vi "Text control 2 v5.1_pump-specific.vi"() -> ()   [LabVIEW 2016]
panel:
  in  "Tab Control":enum32{"Main", "Other parameters"}(tab)
  out "Line running":i32
  out "Total lines":i32
  out "Path":path=path "C:/users/rlp38/09Apr2009LTtesting/test2.txt"
  out "I vs Vg":cluster{"Y data in":dbl[], "X data in":dbl[]}[](graph)
  out "Is max":dbl format="%.2e"
  out "Id max":dbl format="%.2e"
  out "Ig max":dbl format="%.2e"
  out "Imax vs time":cluster{"Y data in":dbl[], "X data in":dbl[]}[](graph)
  out "Imin vs time":cluster{"Y data in":dbl[], "X data in":dbl[]}[](graph)
  out "I vs Vd":cluster{"Y data in":dbl[], "X data in":dbl[]}[](graph)
  in  "Program":string="#-------------------------------------------------------\n# Priming script\n#\n# Version 0.5\n# Author: Dimitrios Simatos\n# Last updated: 2017-10-17\n#-------------------------------------------------------\n# Description\n#\n# This script is designed to prime inlet ports 3, 5 and outlet port 2.\n#-------------------------------------------------------\n# Changes\n#\n# Replaced instances of counterclockwise with clockwise rotation.\n#-------------------------------------------------------\n# Important points\n#\n# Never leave any liquid in the pump to dry after the experiments. If they dry, the residue may block the valve.\n# Always run the cleaning cycle after the experiments.\n# Use clockwise rotation when going up in valve port numbers and vice versa.\n#-------------------------------------------------------\n# Things to do before running the script\n#\n# Set time units to minutes.\n# Set filenames.\n# Replace the tubing, if necessary.\n#-------------------------------------------------------\n# Port connections\n#\n# Port 1: Waste\n# Port 2: Waste\n# Port 3: Ultrapure water\n# Port 4: Nothing\n# Port 5: Phosphate buffer (pH=3.2 - 50 mM)\n# Port 6: Nothing\n#-------------------------------------------------------\n# Pumping cycles and execution time\n#\n# Execution time: 4 x 2 = 8 minutes\n# Ultrapure water must be the last to be pumped through the valve, to wash away residual ions.\n# There are 4 pumping cycles. The first two are small, priming cycles, and the last two are large, cleaning and priming cycles.\n# Each small pumping cycle primes the tubing of each port.\n# The last two cycle prime the tubing of the port containing ultrapure water (port 3) and also pump it through the valve, to clean the valve, the syringe, and prime the tubing of the device port (port 2).\n# The device must be disconnected from the port during the priming procedure.\n#-------------------------------------------------------\n# Volume of liquid needed\n#\n# Volume of liquid needed per small cycle: 200 ul\n# Volume of liquid needed per large cycle: 800 ul\n# Total volume of liquid needed per script run:\n# 200 ul of phosphate buffer (pH=3.2 - 50 mM)\n# 200 + 2 x 800 = 1800 ul of ultrapure water\n#-------------------------------------------------------\n# Parameters\n#\n# Syringe size: 1 ml\n# Step resolution N = 0.01 mm\n# Flow V = 300 pulses/second (6000 ul/min)\n#-------------------------------------------------------\n# Cycle 1: Priming the tubing of the phosphate buffer (pH=3.2 - 50 mM) port (port 5)\npump /1ZR #initialize pump\npump /1Q #query pump\npump /1? #report absolute plunger position\n#pump /1?6 #report valve position\nwait-min 1 #wait 1 minute\npump /1N0R #set step resolution: 0.01 mm\npump /1Q #query pump\npump /1? #report absolute plunger position (the plunger should be at 0)\npump /1?6 #report valve position\nwait 1000 #wait 1 second\npump /1V300R #choose speed: 300 steps/s\npump /1Q #query pump\nwait 1000 #wait 1 second\npump /1O5R #go to port 5, counterclockwise rotation\npump /1Q #query pump\npump /1?6 #report valve position\nwait 1000 #wait 1 second\npump /1A600R #go to absolute position 600 (= draw 200 ul)\n# The position of the plunger depends on the volume of the tubing. The syringe must draw enough liquid to fill the tubing.\nwait 30000 #wait 30 seconds\npump /1Q #query pump\npump /1? #report absolute plunger position (the plunger should have finished moving)\n#pump /1?6 #report valve position\npump /1I1R #switch to port 1, clockwise rotation\npump /1Q #query pump\npump /1?6 #report valve position\npump /1A0R #go to absolute position 0 (= empty syringe)\npump /1Q #query pump\npump /1? #report absolute plunger position (the plunger should be moving to 0)\n#pump /1?6 #report valve position\nwait-min 1 #wait 1 minute\n#-------------------------------------------------------\n# Cycle 2: Priming the tubing of the ultrapure water port (port 3)\n#pump /1ZR #initialize pump\npump /1Q #query pump\npump /1? #report absolute plunger position\npump /1?6 #report valve position\nwait-min 1 #wait 1 minute\npump /1N0R #set step resolution: 0.01 mm\npump /1Q #query pump\npump /1? #report absolute plunger position (the plunger should be at 0)\npump /1?6 #report valve position\nwait 1000 #wait 1 second\npump /1V300R #choose speed: 300 steps/s\npump /1Q #query pump\nwait 1000 #wait 1 second\npump /1I3R #go to port 3, clockwise rotation\npump /1Q #query pump\npump /1?6 #report valve position\nwait 1000 #wait 1 second\npump /1A600R #go to absolute position 600 (= draw 200 ul)\n# The position of the plunger depends on the volume of the tubing. The syringe must draw enough liquid to fill the tubing.\nwait 30000 #wait 30 seconds\npump /1Q #query pump\npump /1? #report absolute plunger position (the plunger should have finished moving)\n#pump /1?6 #report valve position\npump /1O1R #switch to port 1, counterclockwise rotation\npump /1Q #query pump\npump /1?6 #report valve position\npump /1A0R #go to absolute position 0 (= empty syringe)\npump /1Q #query pump\npump /1?6 #report valve position\npump /1? #report absolute plunger position (the plunger should be moving to 0)\n#pump /1?6 #report valve position\nwait-min 1 #wait 1 minute\n#-------------------------------------------------------\n# Cycle 3: Cleaning the syringe and the tubing of device port (port 2) (1/2)\n#pump /1ZR #initialize pump\npump /1Q #query pump\npump /1? #report absolute plunger position\npump /1?6 #report valve position\nwait-min 1 #wait 1 minute\npump /1N0R #set step resolution: 0.01 mm\npump /1Q #query pump\npump /1? #report absolute plunger position (the plunger should be at 0)\npump /1?6 #report valve position\nwait 1000 #wait 1 second\npump /1V300R #choose speed: 300 steps/s\npump /1Q #query pump\nwait 1000 #wait 1 second\npump /1I3R #go to port 3, clockwise rotation\npump /1Q #query pump\npump /1?6 #report valve position\nwait 1000 #wait 1 second\npump /1A2400R #go to absolute position 2400 (= draw 800 ul)\n# The position of the plunger depends on the volume of the tubing. The syringe must draw enough liquid to fill the tubing.\nwait 30000 #wait 30 seconds\npump /1Q #query pump\npump /1? #report absolute plunger position (the plunger should have finished moving)\n#pump /1?6 #report valve position\npump /1O2R #switch to port 2, counterclockwise rotation\npump /1Q #query pump\npump /1?6 #report valve position\npump /1A0R #go to absolute position 0 (= empty syringe)\npump /1Q #query pump\npump /1? #report absolute plunger position (the plunger should be moving to 0)\n#pump /1?6 #report valve position\nwait-min 1 #wait 1 minute\n#-------------------------------------------------------\n# Cycle 4: Cleaning the syringe and the tubing of device port (port 2) (2/2)\n#pump /1ZR #initialize pump\npump /1Q #query pump\npump /1? #report absolute plunger position\npump /1?6 #report valve position\nwait-min 1 #wait 1 minute\npump /1N0R #set step resolution: 0.01 mm\npump /1Q #query pump\npump /1? #report absolute plunger position (the plunger should be at 0)\npump /1?6 #report valve position\nwait 1000 #wait 1 second\npump /1V300R #choose speed: 300 steps/s\npump /1Q #query pump\nwait 1000 #wait 1 second\npump /1I3R #go to port 3, clockwise rotation\npump /1Q #query pump\npump /1?6 #report valve position\nwait 1000 #wait 1 second\npump /1A2400R #go to absolute position 2400 (= draw 800 ul)\n# The position of the plunger depends on the volume of the tubing. The syringe must draw enough liquid to fill the tubing.\nwait 30000 #wait 30 seconds\npump /1Q #query pump\npump /1? #report absolute plunger position (the plunger should have finished moving)\n#pump /1?6 #report valve position\npump /1O2R #switch to port 2, counterclockwise rotation\npump /1Q #query pump\npump /1?6 #report valve position\npump /1A0R #go to absolute position 0 (= empty syringe)\npump /1Q #query pump\npump /1? #report absolute plunger position (the plunger should be moving to 0)\n#pump /1?6 #report valve position\nwait-min 1 #wait 1 minute\n#-------------------------------------------------------"
  out "Command running:":string
  out "Serial port data":string
  out "Elapsed Time":dbl caption="Elapsed Time (s)"
  in  "Units":u16(ring)=1 items=["Seconds", "Minutes", "Hours"]
  in  "Time Offset":dbl caption="Set Start Time (s)"
  in  "Reset":bool
  in  "Auto Reset":bool
  in  "integration time":u32(slide) max=2 step=1 scale=0.0..2.0
  in  "Interrupt run":bool
  out "Absolute plunger position vs time":cluster{"Y data in":dbl[], "X data in":dbl[]}[](graph)
  out "Valve position vs time":cluster{"Y data in":dbl[], "X data in":dbl[]}[](graph)
  in  "Halt pump":bool
  in  "Hard stop pump":bool
  out "Is on":dbl format="%.2e"
  out "Id on":dbl format="%.2e"
  out "Ig on":dbl format="%.2e"
  out "Ion vs time":cluster{"Y data in":dbl[], "X data in":dbl[]}[](graph)
  out "Ioff vs time":cluster{"Y data in":dbl[], "X data in":dbl[]}[](graph)
  out "Ig min":dbl format="%.2e"
  out "Id min":dbl format="%.2e"
  out "Is min":dbl format="%.2e"
  out "Is off":dbl format="%.2e"
  out "Id off":dbl format="%.2e"
  out "Ig off":dbl format="%.2e"
  in  "Gate Range\nmode":u16(ring) items=["Auto", "Limited", "Fixed"]
  in  "Gate Range":u8(slide)=6 max=11 scale=0.0..11.0
  in  "Source/Drain\nRange mode":u16(ring) items=["Auto", "Limited", "Fixed"]
  in  "Source/Drain Range":u8(slide)=6 max=11 scale=0.0..11.0
  in  "Panel Controls":T1={"Emergency Stop"=refnum, "TransGraph Max"=1e-05, "Text/Graph (text=false)"=TRUE} {"TransGraph Max" format="%.2e"}
  in  "Panel Controls 2":T2={"Emergency Stop"=refnum, "TransGraph Max"=1e-05, "Text/Graph (text=false)"=TRUE, "TransGraph Min"=1e-11} {"TransGraph Min" format="%.2e"; "TransGraph Max" format="%.2e"}
  in  "SMU4":cluster{"on/off":bool, "Voltage":dbl} {"Voltage" min=-100.0 max=100.0 format="%.2f"}
  in  "Full Reset":bool
  in  "Standby":T3
  out "error out":errorcluster
  in  "Delay before read (ms)":u32=1000
  in  "byte count":u32=64
  in  "Serial End Mode for Reads":u16(ring)=2 items=["None", "LastBit", "TermChar"]
  in  "Timeout (ms)":u32=10000
  in  "Enable Termination\nChar (T)":bool=TRUE
  in  "Termination char\n(0xA = '\\n' = LF)\n(0xD = '\\r' = CR)":u8=13 format="%.0x"
  in  "flow control":u16(ring) items=["None"=0, "XON/XOFF"=1, "RTS/CTS"=2, "DTR/DSR"=4]
  in  "stop bits":u16(ring)=10 items=["1.0"=10, "1.5"=15, "2.0"=20]
  in  "parity":u16(ring) items=["None", "Odd", "Even", "Mark", "Space"]
  in  "data bits":u16=8 min=5 max=8 step=1
  in  "VISA resource name":refnum<visa-resource-name>="COM6"
  in  "baud rate":u32=9600
  in  "Drain: Compliance":dbl=0.001 format="%.8f"
  in  "Gate: Compliance":dbl=0.001 format="%.8f"
  in  "hold time /s":dbl format="%.2f"
  in  "delay time /s":dbl format="%.2f"
  in  "Integration time (short)":dbl=0.0019 min=8e-05 max=0.0019 step=8e-05 format="%^.0e"
  in  "Integration time (long)":dbl=0.32 min=0.04 max=2.0 step=0.02 format="%.2f"
  in  "Step delay /s":dbl format="%.2f"
  in  "Prefix (transfer)":string="_step_1_ultrapure_H2O_"
  in  "Suffix (transfer)":string="_T.txt"
  in  "Prefix (Imax,Imin,Ion,Ioff)":string="_step_1_ultrapure_H2O_Imax_Imin_Ion_Ioff_vs_time"
  in  "Suffix (Idmax-Idmin)":string=".txt"
  in  "Prefix (output)":string="_step_1_ultrapure_H2O_"
  in  "Suffix (output)":string="_O.txt"
  in  "Prefix (script)":string="_step_1_ultrapure_H2O_script"
  in  "Prefix (serial port log)":string="_step_1_ultrapure_H2O_serial port output"
  in  "Prefix (plunger)":string="_step_1_ultrapure_H2O_plunger_vs_time"
  in  "Suffix (plunger)":string=".txt"
  in  "Prefix (valve)":string="_step_1_ultrapure_H2O_valve_port_vs_time"
  in  "Suffix (valve)":string=".txt"
  in  "Gate":T4={"Gate Start"=0.0, "Gate Stop"=2.0, "Gate Step (linear only)"=1.0, "Gate Compliance"=0.0001, "Gate PComp"=0.0, "Range mode"=0, "Range"=6} {"Range" max=11 scale=0.0..11.0; "Range mode" items=["Auto", "Limited", "Fixed"]; "Gate PComp" format="%^.2e"; "Gate Compliance" format="%^.2e"; "Gate Step (linear only)" format="%^.4e"; "Gate Stop" format="%^.4e"; "Gate Start" format="%^.4e"}
  in  "Drain 2":T5={"Drain Start"=0.0, "Drain Stop"=2.0, "Drain Compliance"=0.0001, "Drain Step"=1.0, "Drain PComp"=0.0, "Range mode"=0, "Range"=6} {"Range" max=11 scale=0.0..11.0; "Range mode" items=["Auto", "Limited", "Fixed"]; "Drain PComp" format="%^.2e"; "Drain Step" format="%^.4e"; "Drain Compliance" format="%^.2e"; "Drain Stop" format="%^.4e"; "Drain Start" format="%^.4e"}
  in  "Timings 2":T6={"integration time"=0, "Short/Long integration time"=0.00064, "hold time (sec)"=0.0, "delay time (sec)"=0.0, "Step Time (0 disables)"=0.0, "sweep method"=0, "Pulse period"=0.005, "Base voltage"=0.0, "Pulse width"=0.0005} {"Pulse width" min=0.0005 max=0.1 step=0.0001 format="%.4f"; "Base voltage" format="%^.4e"; "Pulse period" min=0.005 max=1.0 step=0.0001 format="%.4f"; "sweep method" items=["Continuous", "Pulsed"]; "Step Time (0 disables)" format="%.2f"; "delay time (sec)" format="%.4f"; "hold time (sec)" format="%.4f"; "Short/Long integration time" format="%^.0e"; "integration time" scale=0.0..2.0}
  # "Syntax:\nitime [s|m|l]\ngaterangemode [a|l|f]\ndrainrangemode [a|l|f]\npulsed [on|off] PulsePeriod(sec) PulseBaseVoltage PulseONWidth(sec)\nstandby [on l off]\nwait NumMilliseconds\nwait-min NumMinutes\n# texthere = comment\ntransfer [s|d] VgStart VgStop VgStep VdStart VdStop VdStep\noutput [s|d] VgStart VgStop VgStep VdStart VdStop VdStep\nsample Vg Vd NumSamples Time(s) SampleInterval(s)\nsamplei Idg NumSamples Time(s) SampleInterval(s) VDGcompliance\n100 samples is approximately 13 seconds with medium integration\n# if in doubt use SampleInterval(s) = 0.004\nstressV VG VD IGcompliance IDcompliance Duration(sec)\nstressI IDG VDGcompliance Duration(sec)\nvsu2pulse Bias Duration(s)\npulsedstressV [s|d] VEstop VgON VgOFF Period(s) PulseONwidth(s) Vd\nsample-fpp Vg Vd NumSamples Time\nresample-fpp Vg Vd\ntransfer-fpp [s|d] VgStart VgStop VgStep VdStart VdStop VdStep\noutput-fpp [s|d] VgStart VgStop VgStep VdStart VdStop VdStep\nserial SerialPortCommand\npump SerialPortCommand for the OEM pump\n\nSPM OEM Pump Syntax (<x>: pump number, use 1 if only one pump):\nif the command syntax contains [R], then append the letter R to the command\n/<x>Q: query (a query command should follow each command)\n/<x>Z[R] or /<x>Y[R]: initialize pump\n/<x>N<n>[R] (<n>=0,1): <0> (<1>) microstep 0.01 mm (0.00125 mm) resolution\n/<x>I<n> (<n>=0-6): turn to port number n (clockwise)\n/<x>O<n> (<n>=0-6): turn to port number n (counterclockwise)\n/<x>X: Re-execute last command string\n/<x>G<n>[R] (<n>=0-60000): repeat command sequence (default: 0, 0=loop forever)\n/<x>g: Mark the start of a repeat sequence (max = 10)\n/<x>M<n>[R] (<n>=0-86400000): delay command execution by n milliseconds\n/<x>H: Halt; Pause the sequence after finishing the current move\n/<x>T: Hardstop; Interrupt the current move and suppress it from the sequence\n/<x>A<n>[R] (<n>=0-3000 with N=0, 0-24000 with N=1): absolute position\n/<x>P<n>[R] (<n>=0-3000 with N=0, 0-24000 with N=1): relative pickup\n/<x>D<n>[R] (<n>=0-3000 with N=0, 0-24000 with N=1): relative dispense\n/<x>V<n>[R] (<n>=1-1600 default: 150): set peak speed (pulses/sec)\nNOTE: The lowest speed limit is 1 pulse/sec, not 5, as the manual states.\n/<x>S<n>[R] (<n>=10-40 default: 22): set speed (NOT in pulses/sec, look in manual)\nNOTE: When controlled with absolute position, one does not need to pay special attention to the syringe that is mounted on the pump.\nWithdraw from lower stage (ports 3, 5), dispense from higher stage (ports 2, 4, 6).\nConnect Port 1 to waste."
  # "Time"
  # "1\n2\n3\n4\n5\n6\n7\n8\n9\n10\n11\n12\n13\n14\n15\n16\n17\n18\n19\n20"
  # "Serial port settings"
  # "Filename settings"
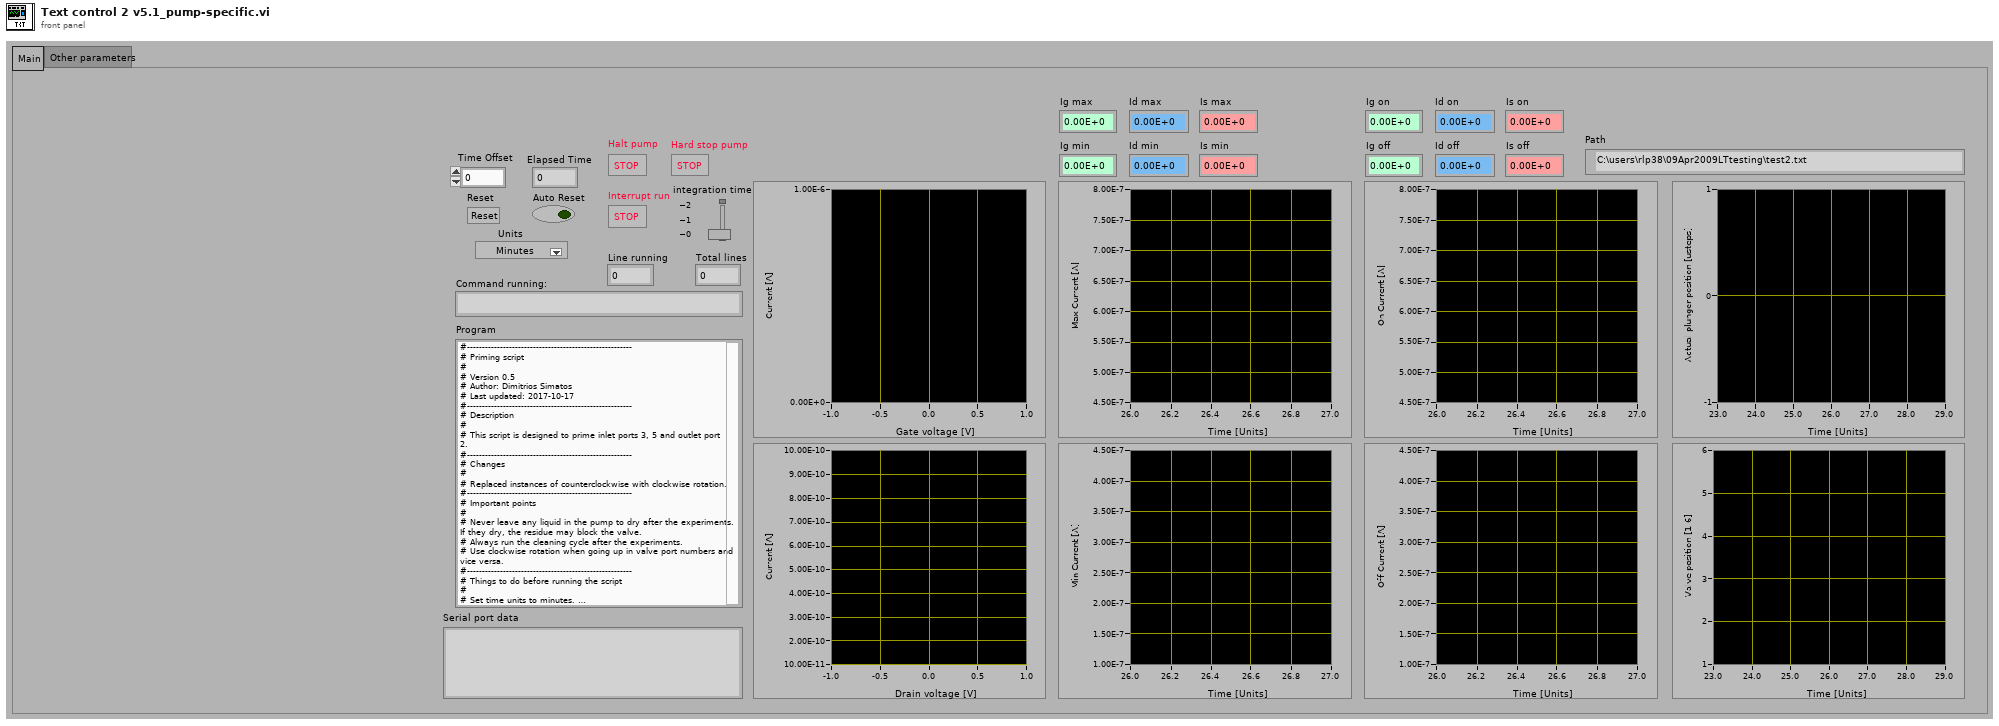
[diagram p1: front panel]
types:
  T1 = cluster{"Emergency Stop":refnum<vi>, "TransGraph Max":dbl, "Text/Graph (text=false)":bool}
  T2 = cluster{"Emergency Stop":refnum<vi>, "TransGraph Max":dbl, "Text/Graph (text=false)":bool, "TransGraph Min":dbl}
  T3 = cluster{"Gate Standby":bool, "Drain Standby":bool}
  T4 = cluster{"Gate Start":dbl, "Gate Stop":dbl, "Gate Step (linear only)":dbl, "Gate Compliance":dbl, "Gate PComp":dbl, "Range mode":u16, "Range":u8}
  T5 = cluster{"Drain Start":dbl, "Drain Stop":dbl, "Drain Compliance":dbl, "Drain Step":dbl, "Drain PComp":dbl, "Range mode":u16, "Range":u8}
  T6 = cluster{"integration time":u32, "Short/Long integration time":dbl, "hold time (sec)":dbl, "delay time (sec)":dbl, "Step Time (0 disables)":dbl, "sweep method":u16, "Pulse period":dbl, "Base voltage":dbl, "Pulse width":dbl}
  T7 = enum16{"open", "replace", "create", "open or create", "replace or create", "replace or create with confirmation"}
  T8 = cluster{"V2 Start":dbl, "V2 Step":dbl, "Number of points":i32}
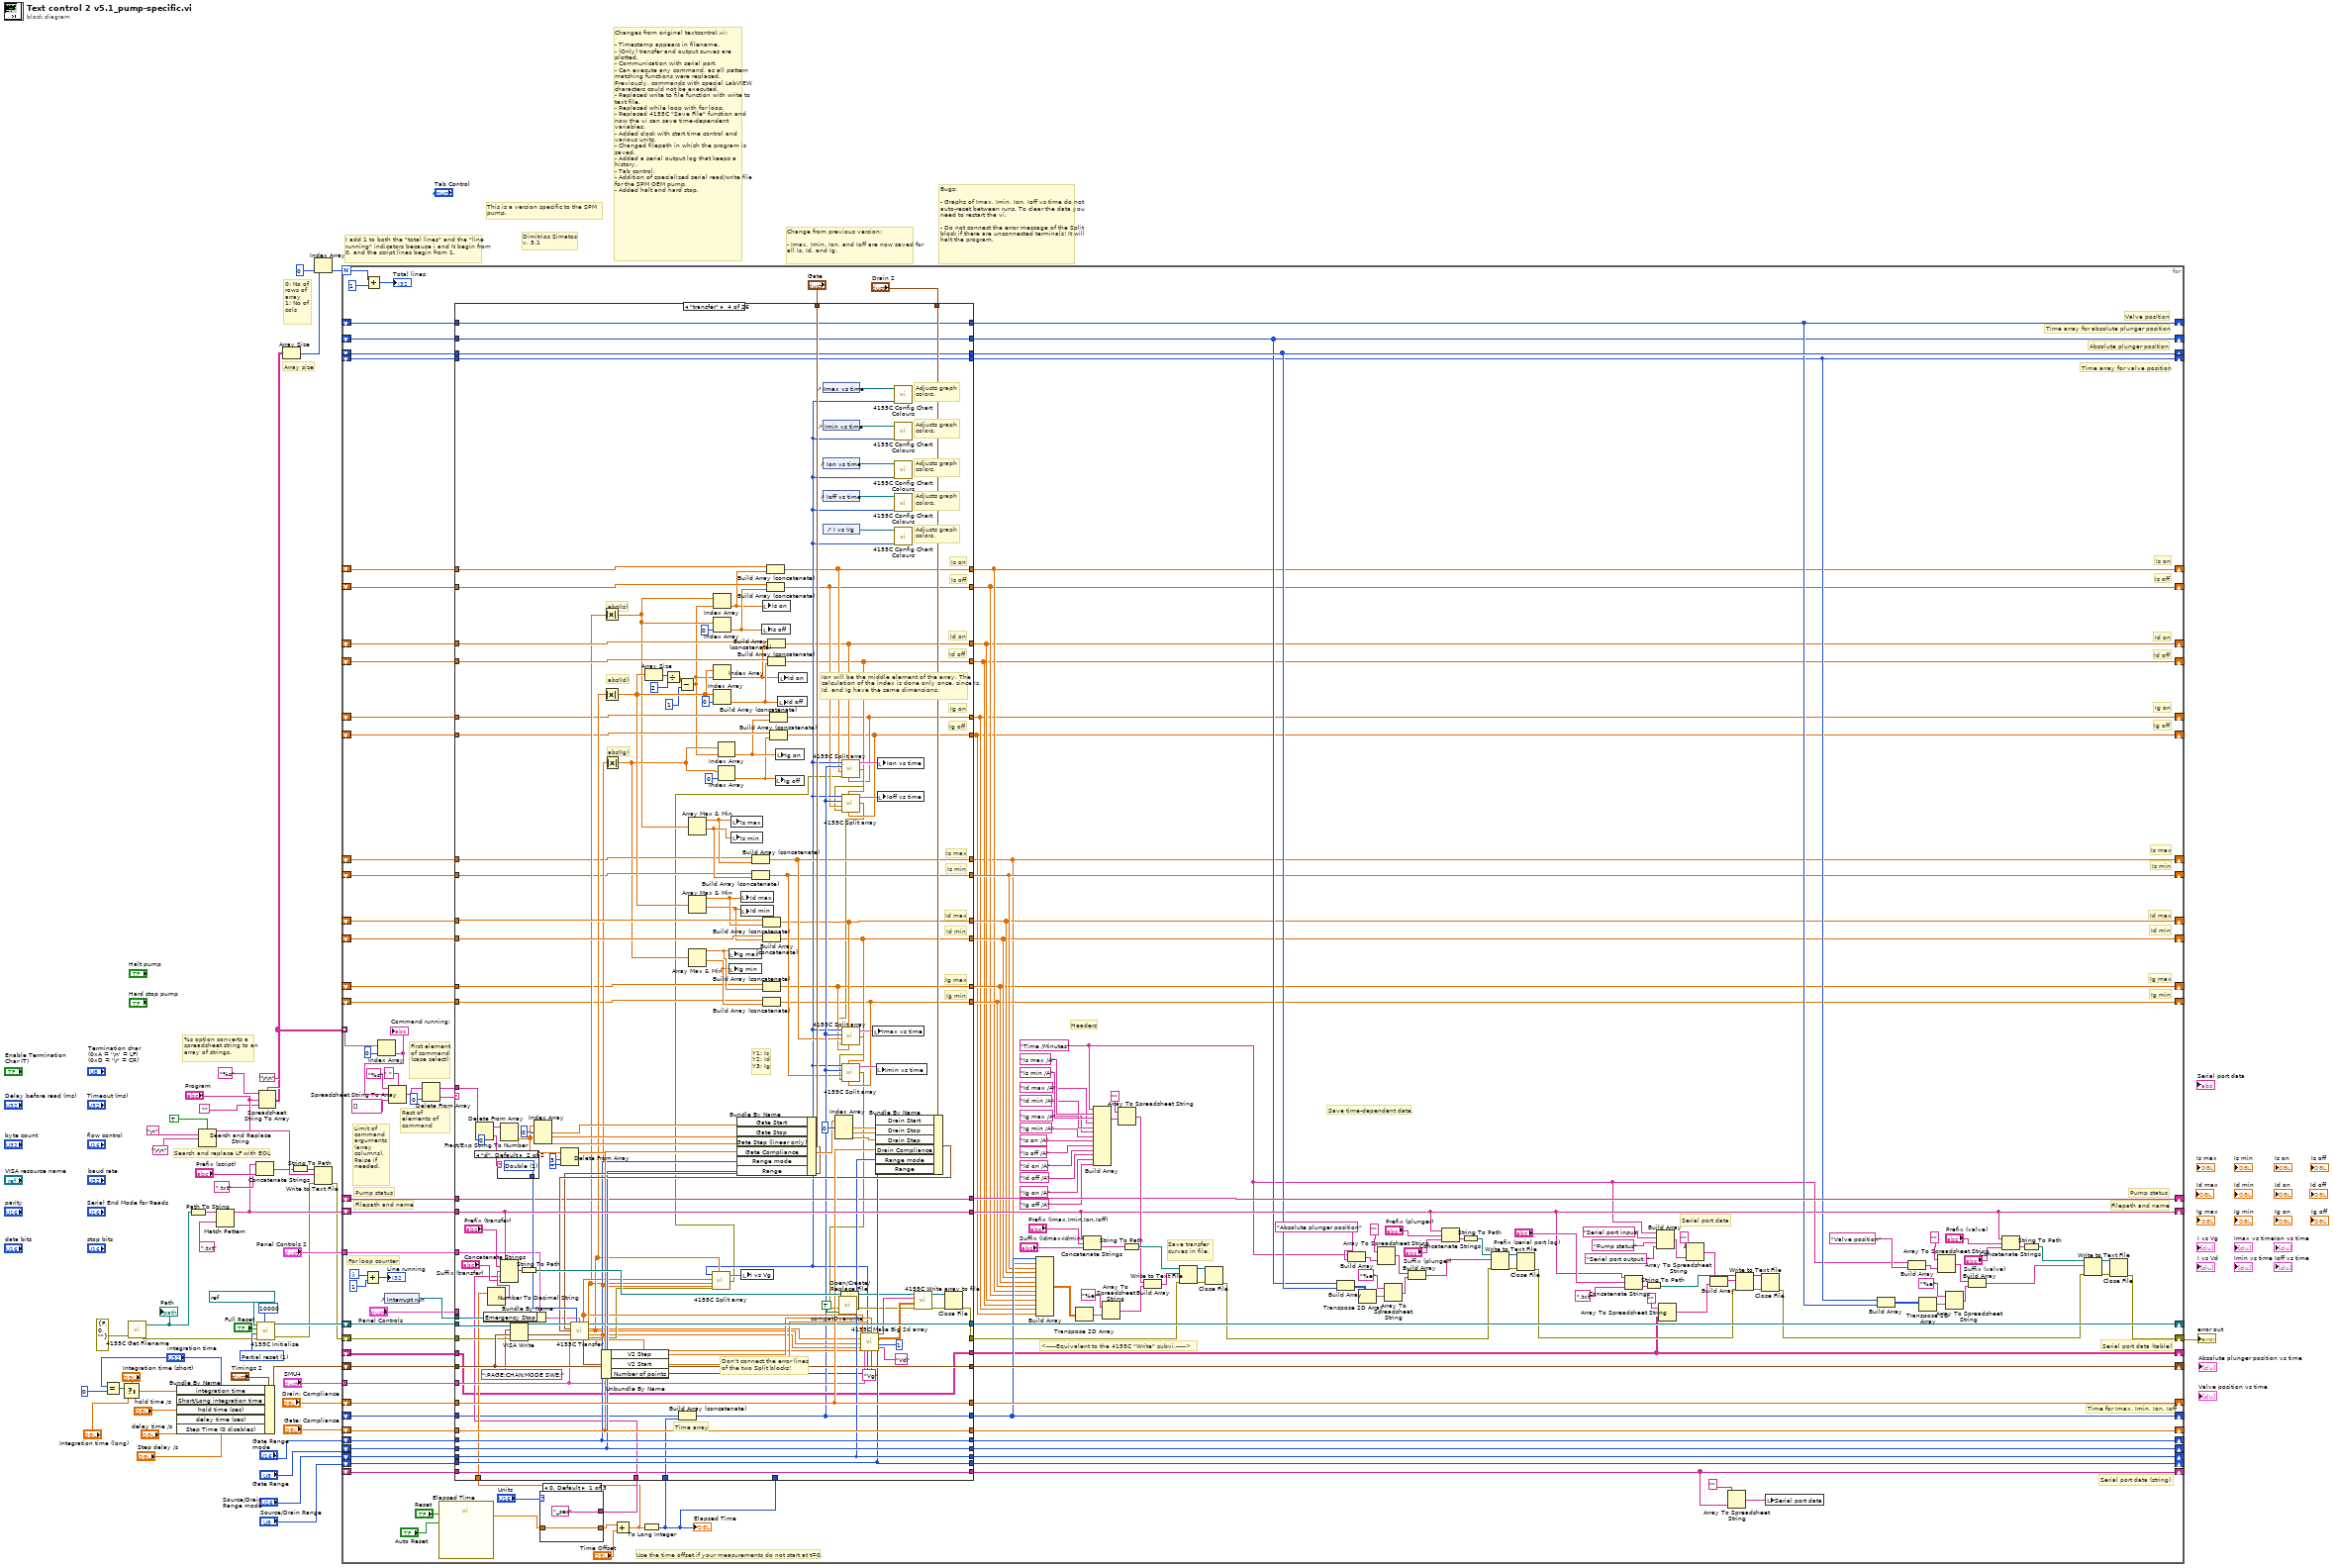
[diagram p0: block diagram]
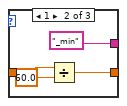
[diagram p2: hidden frame]
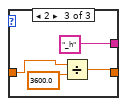
[diagram p3: hidden frame]
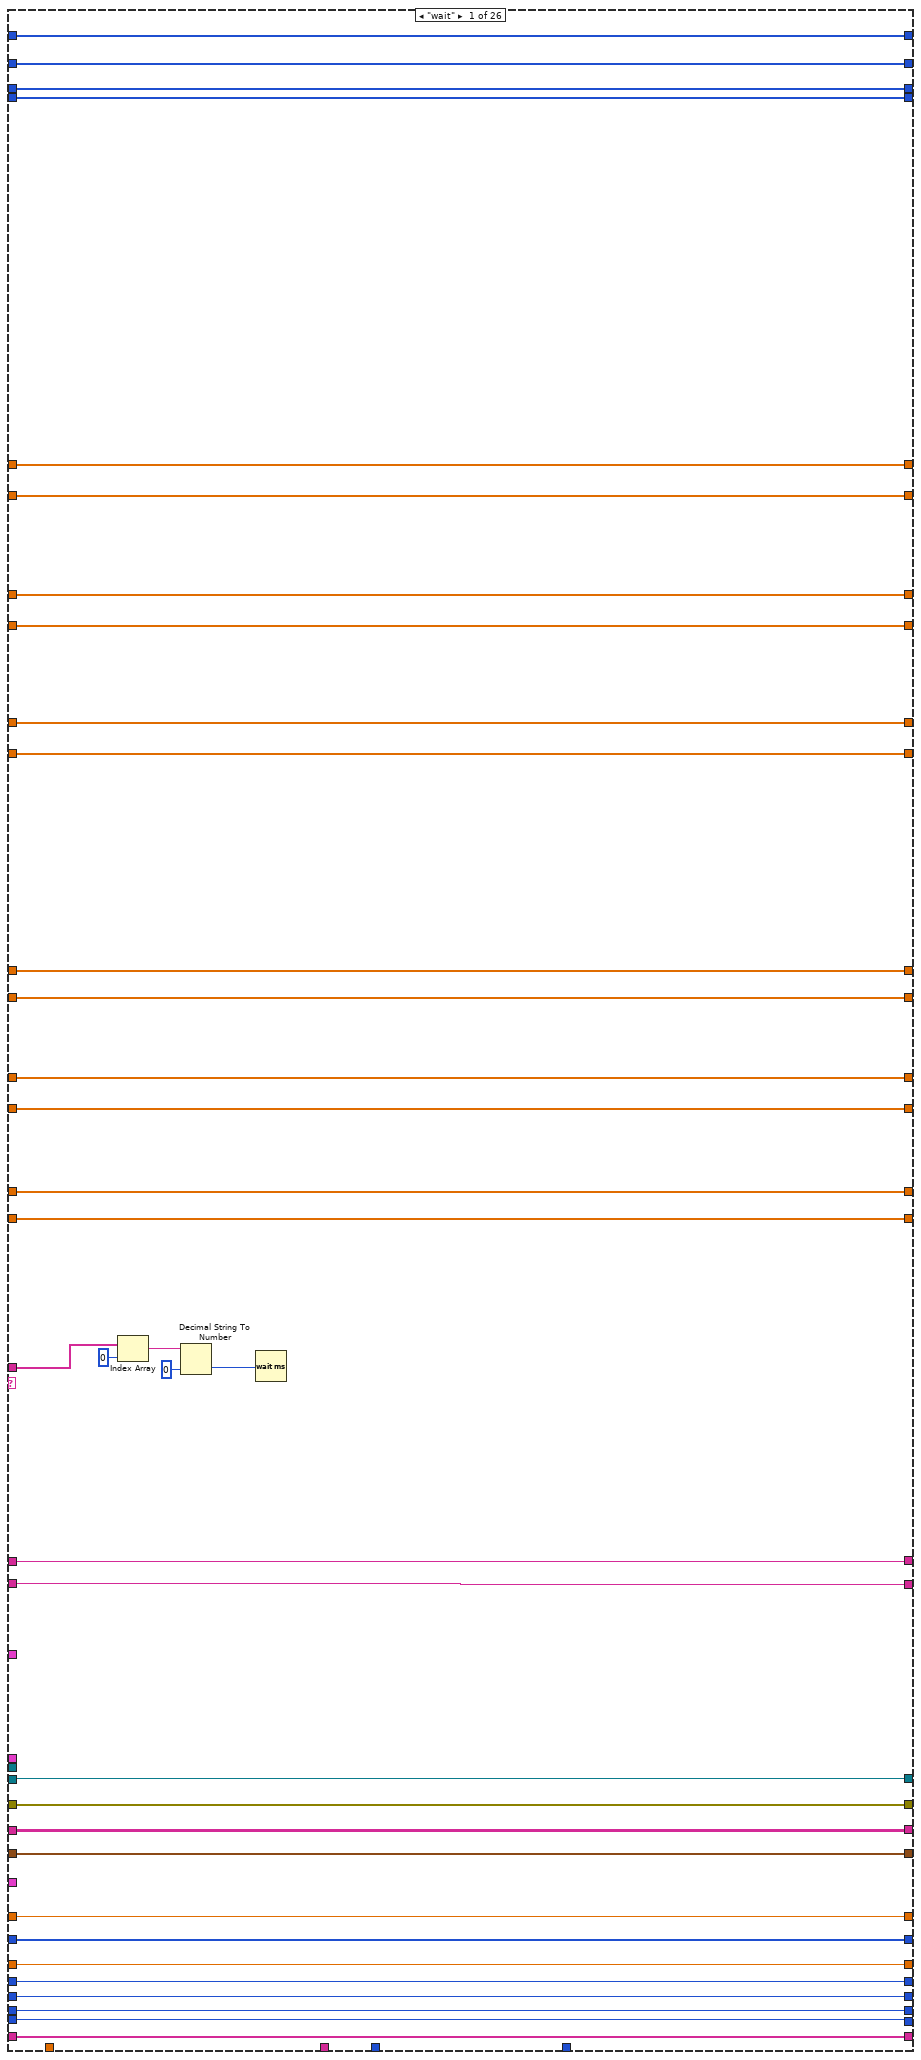
[diagram p4: hidden frame]
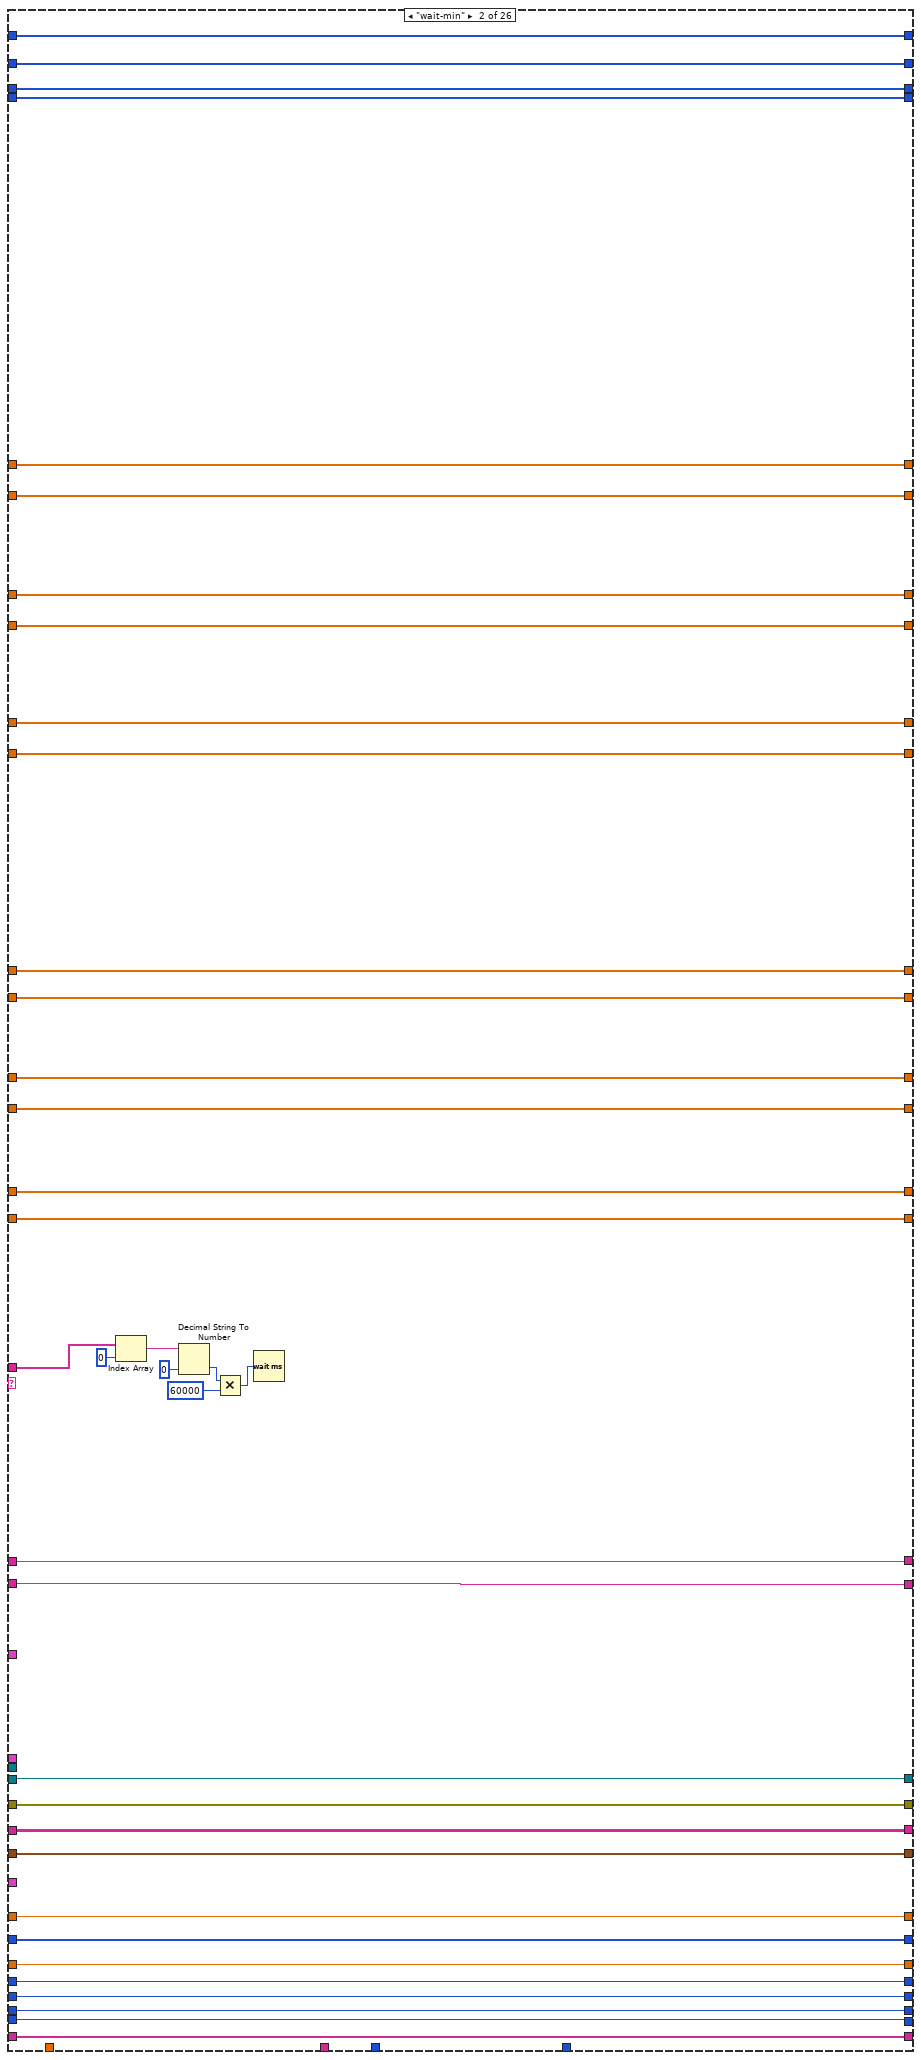
[diagram p5: hidden frame]
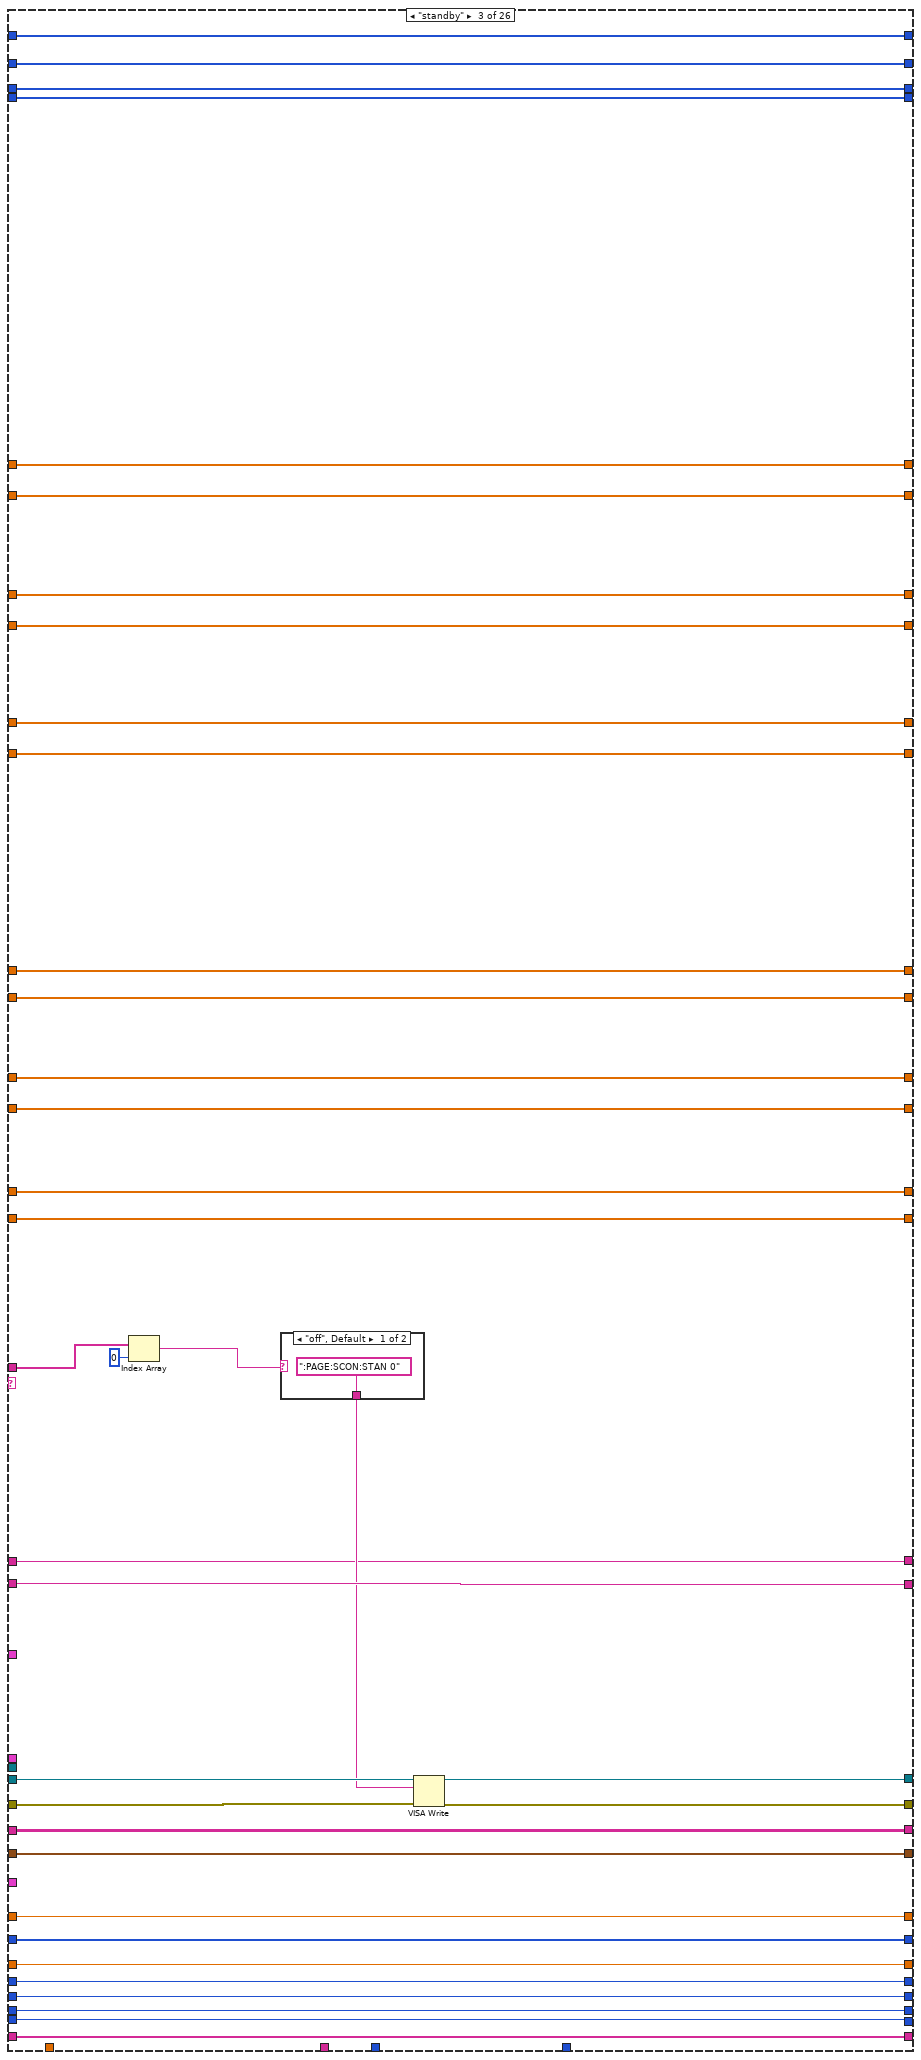
[diagram p6: hidden frame]
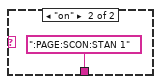
[diagram p7: hidden frame]
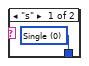
[diagram p8: hidden frame]
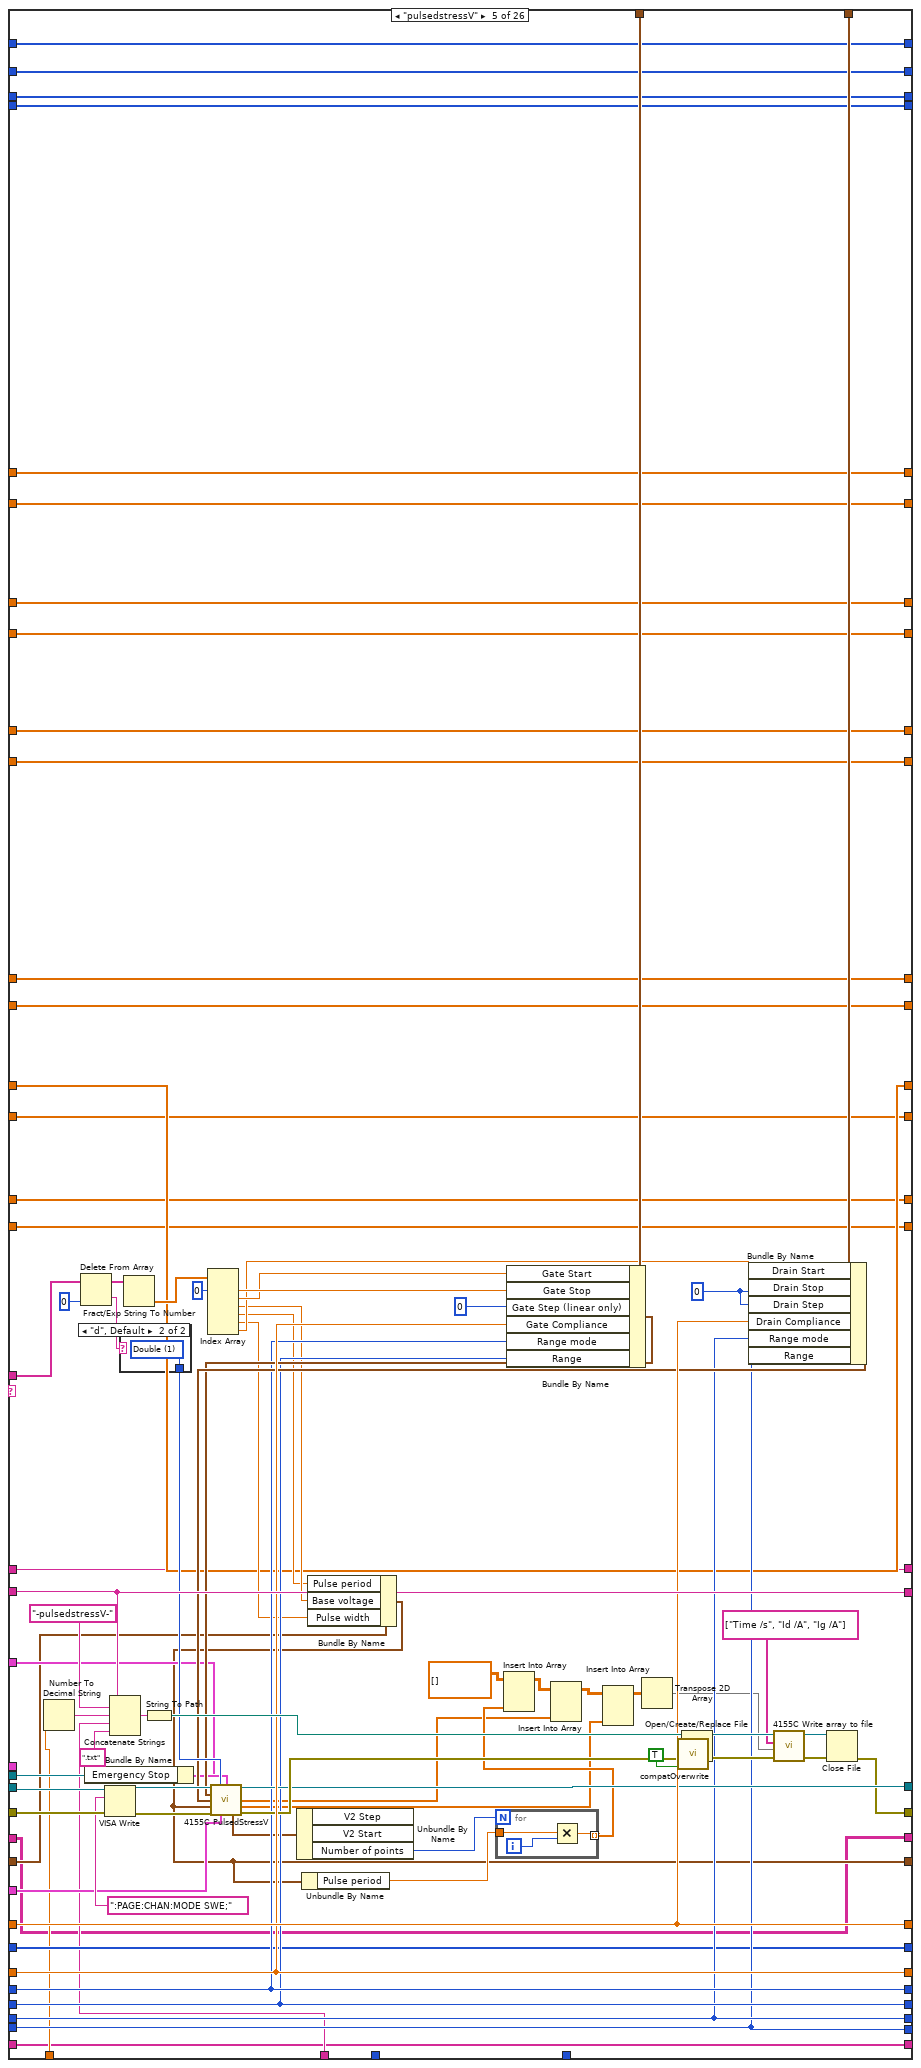
[diagram p9: hidden frame]
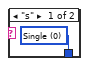
[diagram p10: hidden frame]
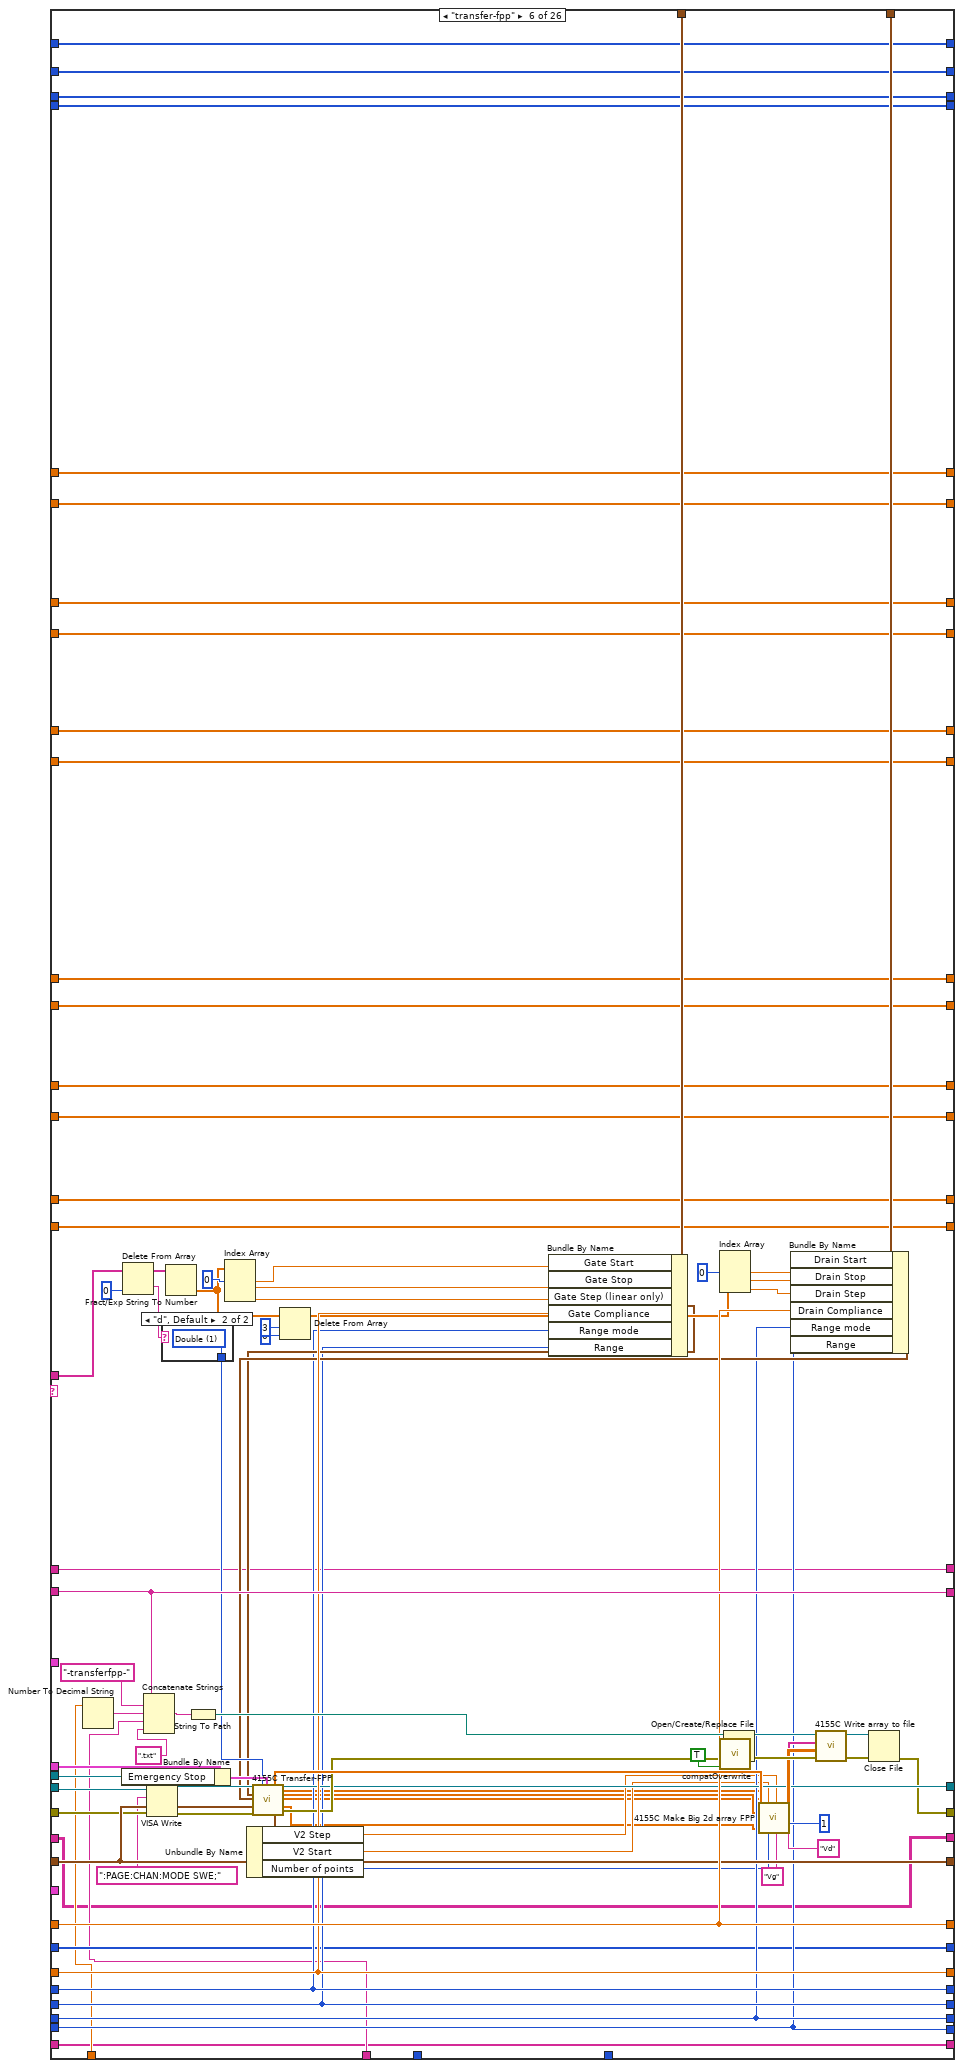
[diagram p11: hidden frame]
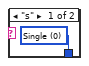
[diagram p12: hidden frame]
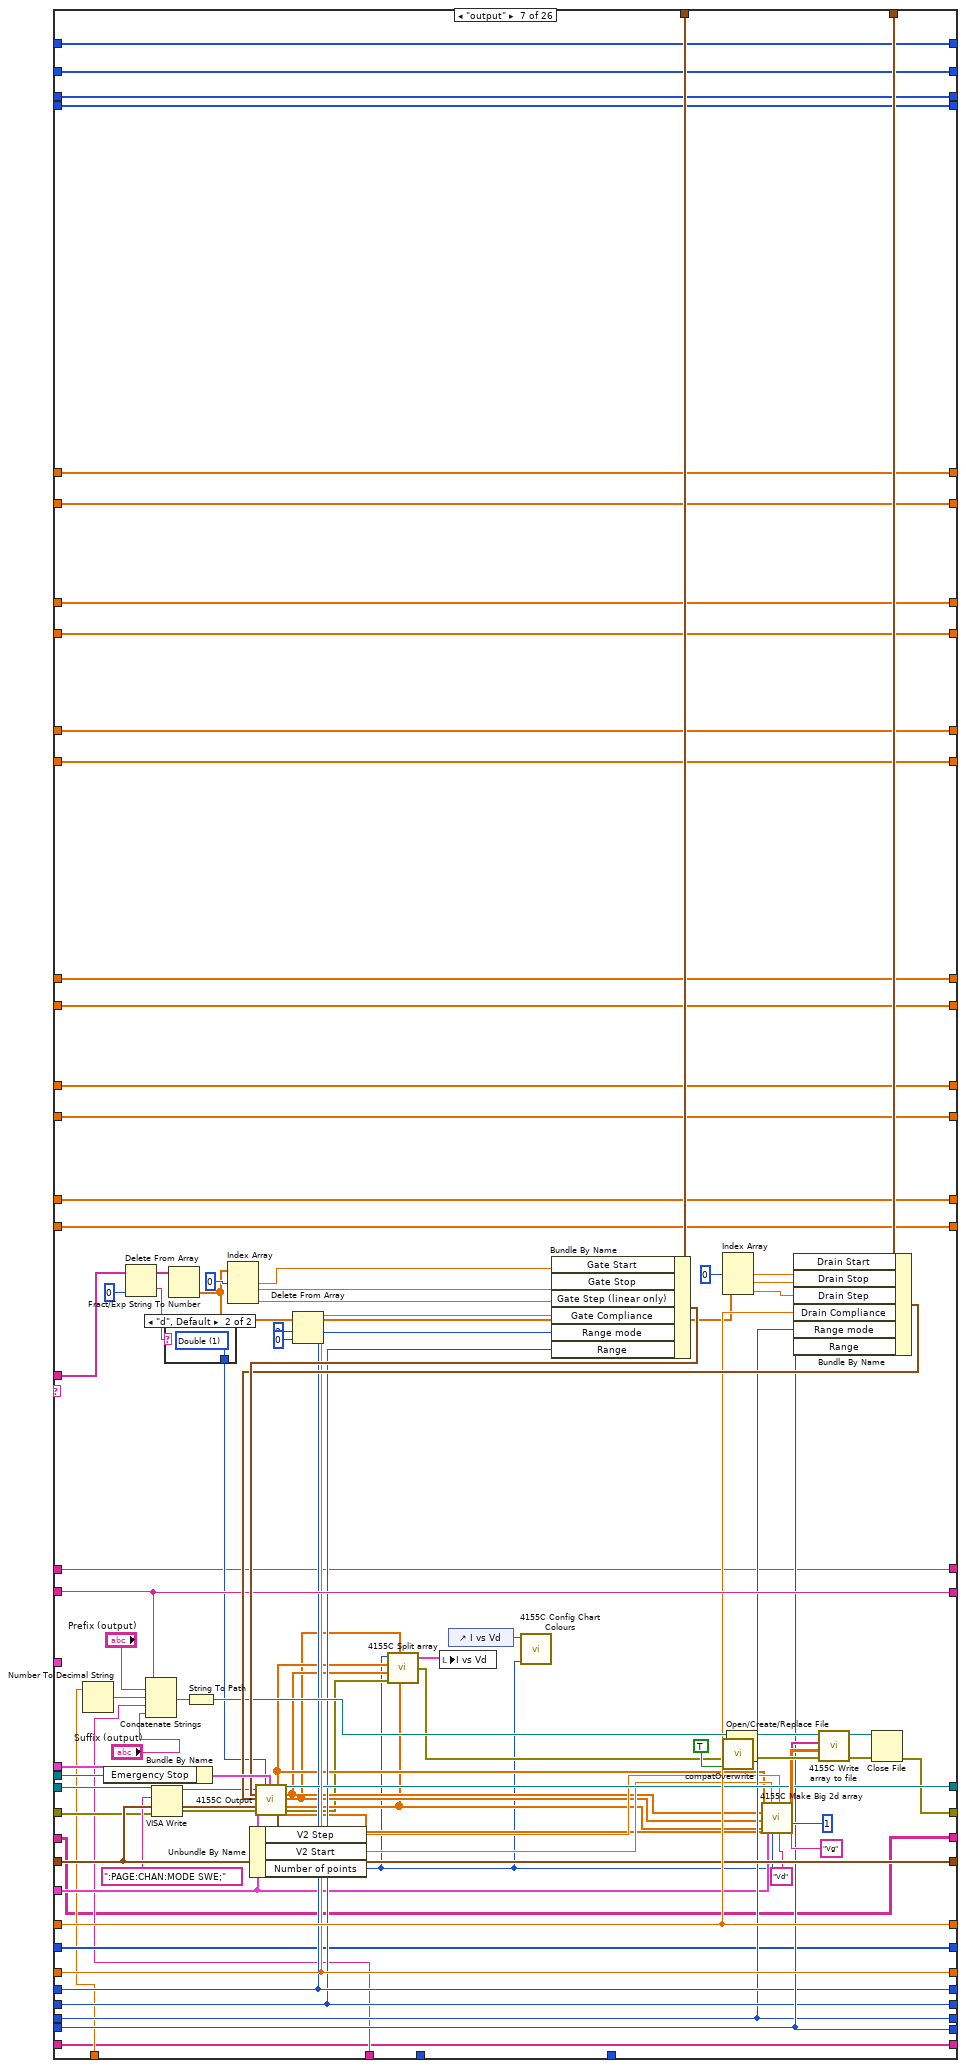
[diagram p13: hidden frame]
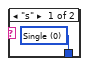
[diagram p14: hidden frame]
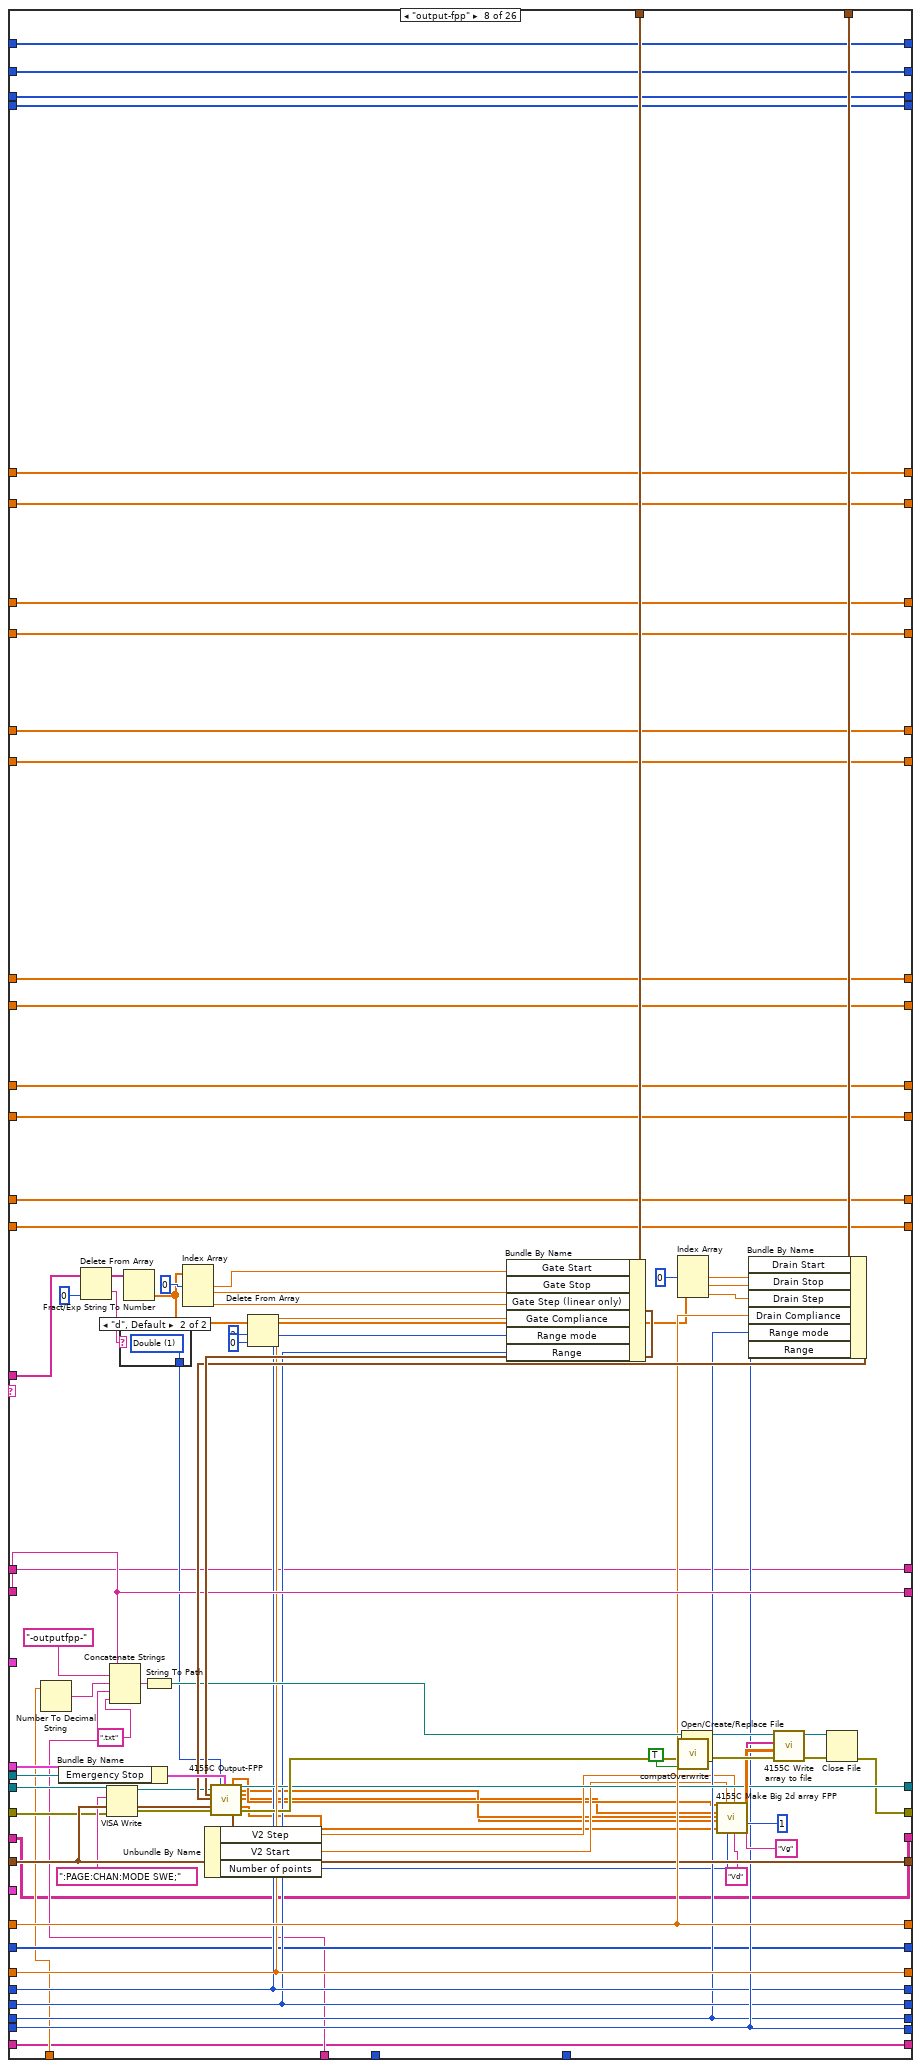
[diagram p15: hidden frame]
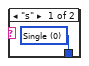
[diagram p16: hidden frame]
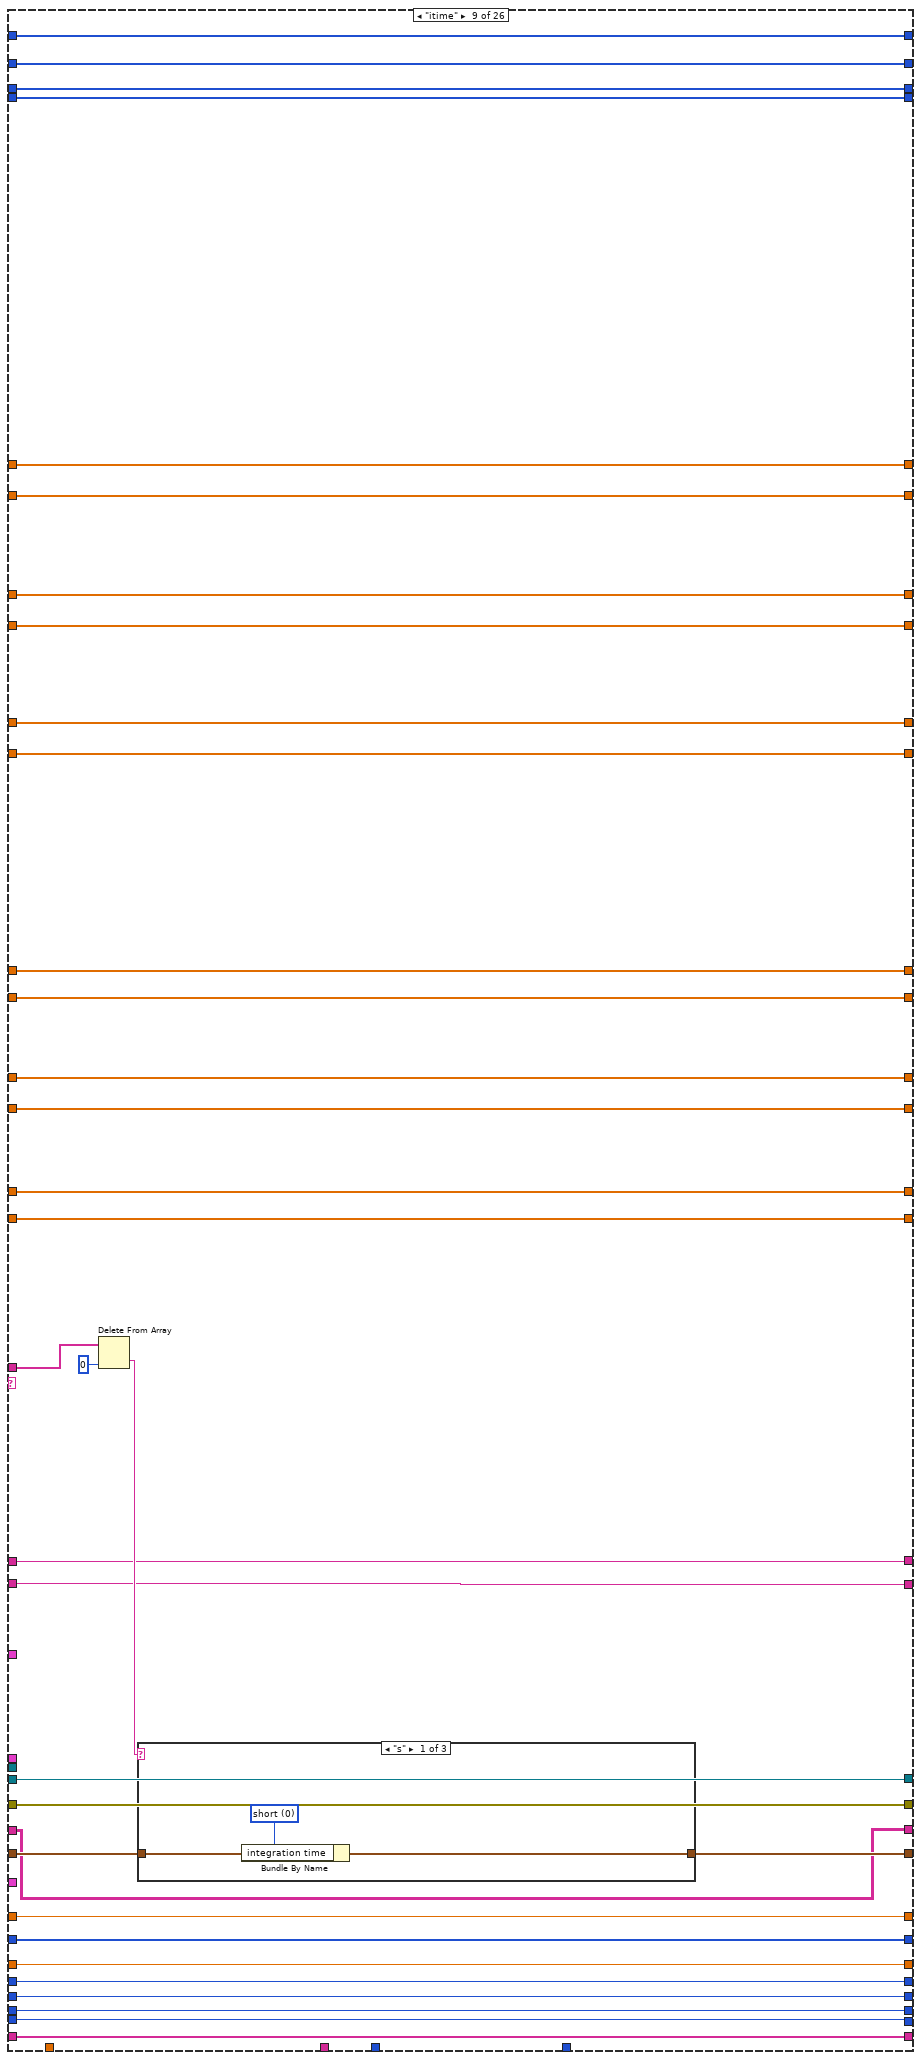
[diagram p17: hidden frame]
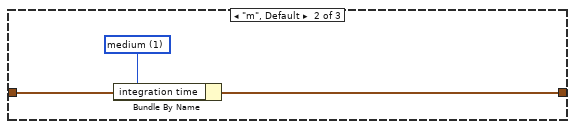
[diagram p18: hidden frame]
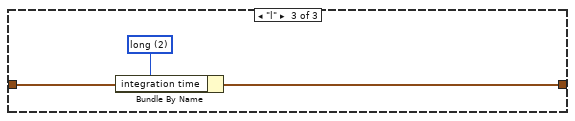
[diagram p19: hidden frame]
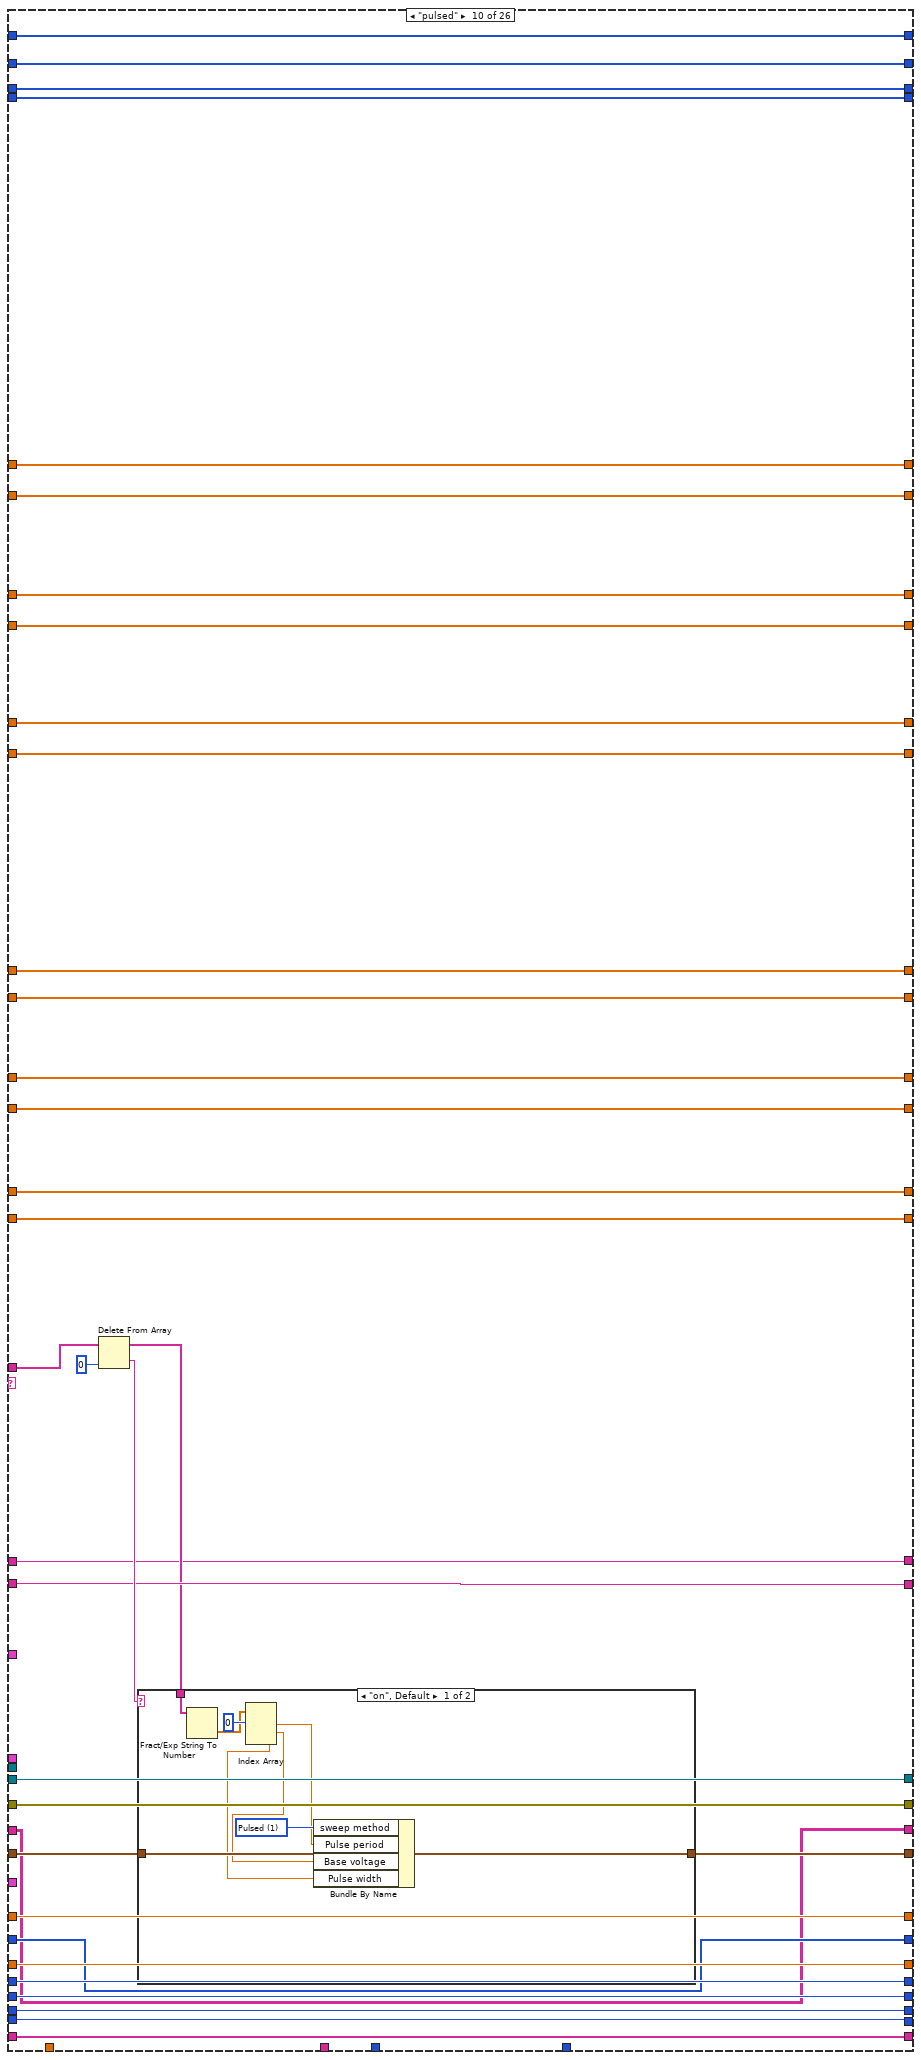
[diagram p20: hidden frame]
diagram:
  w40 = u16 1 items=["Reset All", "Partial reset"] ("Type of reset")
  # "Change from previous version:\n\n- Imax, Imin, Ion, and Ioff are now saved for all Is, Id, and Ig."
  # "This is a version specific to the SPM pump."
  # "I add 1 to both the \"total lines\" and the \"line running\" indicators because i and N begin from 0, and the script lines begin from 1."
  # "Bugs:\n\n- Graphs of Imax, Imin, Ion, Ioff vs time do not auto-reset between runs. To clear the data you need to restart the vi.\n\n- Do not connect the error message of the Split block if there are unconnected terminals! It will halt the program."
  # "Array size"
  # "%s option converts a spreadsheet string to an array of strings."
  # "0: No of rows of array\n1: No of cols"
  # "Dimitrios Simatos\nv. 5.1"
  # "Changes from original textcontrol.vi:\n\n- Timestamp appears in filename.\n- (Only) transfer and output curves are plotted.\n- Communication with serial port.\n- Can execute any command, as all pattern matching functions were replaced. Previously, commands with special LabVIEW characters could not be executed.\n- Replaced write to file function with write to text file.\n- Replaced while loop with for loop.\n- Replaced 4155C \"Save File\" function and now the vi can save time-dependent variables.\n- Added clock with start time control and various units.\n- Changed filepath in which the program is saved.\n- Added a serial output log that keeps a history.\n- Tab control.\n- Addition of specialized serial read/write file for the SPM OEM pump.\n- Added halt and hard stop."
  # "Search and replace LF with EOL"
  n1 = Equal?(x="integration time", y=u32 0) -> (x = y?=w44:bool)
  n2 = Select(t="Integration time (short)", s=w44, f="Integration time (long)") -> (s? t:f=w48:dbl)
  n3 = call "4155C Get Filename.vi"("error in (no error)"=errorcluster {"status"=FALSE, "code"=0, "source"=""}) -> ("error out"=w35:errorcluster, "path"=w10:path)  [unwired: 2 in, 1 out]
  "Path" <- w10
  n4 = Bundle By Name(cluster="Timings 2", "integration time"="integration time", "Short/Long integration time"=w48, "hold time (sec)"="hold time /s", "delay time (sec)"="delay time /s", "Step Time (0 disables)"="Step delay /s") -> (w33:T6)
  n5 = Path To String(path=w10) -> (string=w11:string)
  n6 = Search and Replace String(replace all?=TRUE ("replace all? (F)"), input string="Program", search string="\n", replace string="\r\n") -> (result string=w23:string)  [unwired: 4 in, 3 out]
  n7 = Match Pattern(string=w11, regular expression=".txt") -> (before substring=w5:string)  [unwired: 1 in, 3 out]
  n8 = Concatenate Strings(w5, "Prefix (script)", ".txt" ("regular expression")) -> (w4:string)
  n9 = call "4155C Initialise.vi"("VISA resource name in"=refnum<visa-resource-name> "GPIB0::14::INSTR", "Reset"="Full Reset", "Type of reset"=w40, "error in (no error)"=w35, "VISA Timeout Value"=u32 10000) -> ("VISA Resource Name out"=w34:refnum<visa-resource-name>, "error out"=w2:errorcluster)
  n10 = Spreadsheet String To Array(delimiter (Tab)="\r\n", format string="%s", spreadsheet string="Program", array type (2D Dbl)="") -> (array=w14:string[][])
  n11 = Array Size(array=w14) -> (size(s)=w18:i32[])
  n12 = String To Path(string=w4) -> (path=w3:path)
  n13 = Index Array(array=w18, index=0) -> (element=w16:i32)
  n14 = Write to Text File(file (use dialog)=w3, text=w23, error in=w2) -> (error out=w1:errorcluster)  [unwired: 1 in, 2 out]
  n15 = for {
    N: w16 -> [w158]
    tunnel: "SMU4" -> [w196]
    shift-left: "Source/Drain Range" -> [w201]
    shift-right: [w197] -> _
    shift-left: "Source/Drain\nRange mode" -> [w202]
    shift-right: [w198] -> _
    shift-left: "Gate Range" -> [w203]
    shift-right: [w199] -> _
    shift-left: "Gate Range\nmode" -> [w204]
    shift-right: [w200] -> _
    shift-left: "Gate: Compliance" -> [w213]
    shift-right: [w209] -> _
    shift-left: "Drain: Compliance" -> [w214]
    shift-right: [w210] -> _
    shift-left: w33 -> [w215]
    shift-right: [w211] -> _
    shift-left: w1 -> [w216]
    shift-right: [w98] -> w9
    shift-left: w34 -> [w217]
    shift-right: [w212] -> _
    shift-left: w5 -> [w218]
    shift-right: [w102] -> _
    tunnel: "Panel Controls 2" -> [w195]
    shift-right: [w60] -> _
    shift-left: _ -> [w194]
    shift-right: [w124] -> _
    shift-left: _ -> [w190]
    tunnel: w14 -> [w189] mode=indexing
    shift-right: [w59] -> _
    shift-left: _ -> [w164]
    shift-right: [w92] -> _
    shift-left: _ -> [w150]
    shift-right: [w125] -> _
    shift-left: _ -> [w143]
    shift-right: [w104] -> _
    shift-left: _ -> [w142]
    shift-right: [w141] -> _
    shift-left: _ -> [w140]
    shift-right: [w97] -> _
    shift-left: _ -> [w121]
    shift-right: [w96] -> _
    shift-left: _ -> [w103]
    shift-right: [w93] -> _
    shift-left: _ -> [w95]
    shift-right: [w53] -> _
    shift-left: _ -> [w81]
    shift-right: [w54] -> _
    shift-left: _ -> [w80]
    shift-right: [w58] -> _
    shift-left: _ -> [w69]
    shift-right: [w57] -> _
    shift-left: _ -> [w68]
    shift-right: [w51] -> _
    shift-left: _ -> [w67]
    shift-right: [w61] -> _
    shift-left: _ -> [w66]
    shift-right: [w52] -> _
    shift-left: _ -> [w65]
    shift-right: [w50] -> _
    shift-left: _ -> [w64]
    shift-right: [w56] -> _
    shift-left: _ -> [w63]
    shift-right: [w55] -> _
    shift-left: _ -> [w62]
    i -> [w153]
    w83 = "Time /Minutes" ("element")
    # "Is off"
    # "Is on"
    # "Ig off"
    # "Ig on"
    # "Is min"
    # "Is max"
    # "Ig min"
    # "Ig max"
    # "Id min"
    # "Id max"
    # "Id off"
    # "Id on"
    # "Pump status"
    # "Filepath and name"
    # "Pump status"
    # "Limit of command arguments (array columns). Raise if needed."
    # "Serial port data (string)"
    # "Serial port data (table)"
    # "Time array for valve position"
    # "Time array for absolute plunger position"
    # "Valve position"
    # "Absolute plunger position"
    # "Serial port data"
    # "For loop counter"
    # "<-----Equivalent to the 4155C \"Write\" subvi.----->"
    # "Headers"
    # "Save transfer curves in file."
    # "Filepath and name"
    # "Save time-dependent data."
    # "Use the time offset if your measurements do not start at t=0."
    # "Time for Imax, Imin, Ion, Ioff"
    # "Rest of elements of command"
    # "First element of command\n(case select)"
    n16 = Add(x=w153, y=1) -> (x+y=→"Line running":i32)
    n17 = Add(x=w158, y=1) -> (x+y=→"Total lines":i32)
    n18 = Index Array(array=w189, index=0 ("line index")) -> (element=w184:string)
    "Command running:" <- w184
    n19 = control-ref of="Interrupt run"() -> (w208:refnum<vi>)
    n20 = Spreadsheet String To Array(delimiter (Tab)=" ", format string="%s", spreadsheet string=w184, array type (2D Dbl)=string[] []) -> (array=w182:string[])
    n21 = Delete From Array(array=w182, index=0) -> (deleted portion=w82:string, array with subset deleted=w181:string[])  [unwired: 1 in]
    n22 = call "Elapsed Time"("Reset"="Reset", "Auto Reset"="Auto Reset") -> ("Elapsed Time (s)"=w191:dbl)  [unwired: 10 in, 7 out]
    n23 = case shown="0, Default" "Units" {
      tunnel: ["_sec" "_min" "_h"] -> w192
      tunnel: [w219 w223 w226] -> w160
      tunnel: w191 -> [w219 w222 w227]
      frame 0, Default {
      }
      frame 1 {
        n24 = Divide(x=w222, y=60.0) -> (x/y=w223:dbl)
      }
      frame 2 {
        n25 = Divide(x=w227, y=3600.0) -> (x/y=w226:dbl)
      }
    }
    n26 = Add(x=w160, y="Time Offset") -> (x+y=w159:dbl)
    n27 = To Long Integer(number=w159) -> (32bit integer=w122:i32)
    "Elapsed Time" <- w122
    n28 = case shown="\"transfer\"" w82 {
      tunnel: w181 -> [w263 w300 w336 w467 w491 w636 w729 w817 w873 w917 w962 w1005 w1044 w1076 _ _ w1234 w1313 _ w1414 w1476 w1536 w1624 w1704 w1742 w1811]
      tunnel: w218 -> [w258 w296 w334 w474 w556 w644 w736 w825 w862 w906 w954 w998 w1038 w1069 w1106 w1166 w1212 w1295 w1344 w1401 w1463 w1524 w1618 w1700 w1744 w1813]
      tunnel: w217 -> [w257 w295 w325 w445 w541 w613 w705 w793 w863 w907 w955 w999 w1039 w1070 w1111 w1168 w1240 w1319 w1348 w1420 w1482 w1542 w1630 w1658 w1748 w1817]
      tunnel: w216 -> [w256 w294 w324 w444 w540 w612 w702 w790 w864 w908 w956 w1000 w1040 w1071 w1110 w1139 w1239 w1318 w1347 w1419 w1481 w1541 w1629 w1657 w1747 w1816]
      tunnel: w215 -> [w255 w293 w333 w470 w516 w640 w732 w821 w872 w916 w953 w997 w1037 w1068 w1109 w1163 w1203 w1287 w1353 w1394 w1456 w1517 w1617 w1699 w1749 w1818]
      tunnel: w214 -> [w254 w292 w332 w472 w554 w642 w734 w823 w871 w915 w961 w1004 w1043 w1075 w1108 w1148 w1238 w1317 w1356 w1418 w1480 w1540 w1628 w1708 w1750 w1819]
      tunnel: w213 -> [w253 w291 w331 w471 w553 w641 w733 w822 w870 w914 w960 w1003 w1042 w1074 w1107 w1149 w1213 w1296 w1355 w1402 w1464 w1525 w1619 w1701 w1752 w1820]
      tunnel: [w257 w295 w323 w469 w551 w638 w731 w819 w863 w907 w955 w999 w1039 w1070 w1111 w1168 w1204 w1269 w1346 w1395 w1457 w1518 w1570 w1660 w1748 w1817] -> w212
      tunnel: [w256 w294 w322 w468 w550 w637 w730 w818 w864 w908 w956 w1000 w1040 w1071 w1110 w1138 w1214 w1270 w1345 w1403 w1465 w1526 w1569 w1659 w1746 w1815] -> w120
      tunnel: [w255 w293 w333 w470 w512 w640 w732 w821 w865 w909 w953 w997 w1037 w1068 w1109 w1163 w1203 w1287 w1353 w1394 w1456 w1517 w1617 w1699 w1749 w1818] -> w211
      tunnel: [w254 w292 w332 w472 w554 w642 w734 w823 w871 w915 w961 w1004 w1043 w1075 w1108 w1148 w1238 w1317 w1356 w1418 w1480 w1540 w1628 w1708 w1750 w1819] -> w210
      tunnel: [w253 w291 w331 w471 w553 w641 w733 w822 w870 w914 w960 w1003 w1042 w1074 w1107 w1149 w1213 w1296 w1355 w1402 w1464 w1525 w1619 w1701 w1752 w1820] -> w209
      tunnel: [w258 w296 w334 w474 w556 w644 w736 w825 w862 w906 w954 w998 w1038 w1069 w1106 w1166 w1212 w1295 w1344 w1401 w1463 w1524 w1618 w1700 w1744 w1813] -> w102
      tunnel: w208 -> [_ _ _ w477 w560 w649 w740 w829 _ _ _ _ _ _ _ _ w1209 w1292 _ w1400 w1462 w1523 w1590 w1676 _ _]
      tunnel: "Gate" -> [_ _ _ w454 w544 w623 w716 w804 _ _ _ _ _ _ _ _ _ _ _ _ _ _ _ _ _ _]
      tunnel: "Drain 2" -> [_ _ _ w453 w543 w622 w715 w803 _ _ _ _ _ _ _ _ _ _ _ _ _ _ _ _ _ _]
      tunnel: "Panel Controls" -> [_ _ _ _ _ w621 w714 w802 _ _ _ _ _ _ _ _ _ _ _ _ _ _ _ _ _ _]
      tunnel: w204 -> [w252 w290 w330 w438 w534 w606 w700 w788 w869 w913 _ w996 w1036 w1067 w1105 w1150 w1199 w1283 w1349 w1390 w1452 w1513 w1613 w1695 w1753 w1821]
      tunnel: w203 -> [w251 w289 w329 w437 w533 w605 w699 w787 w868 w912 w959 _ w1027 w1073 w1104 w1151 w1200 w1284 w1350 w1391 w1453 w1514 w1614 w1696 w1754 w1822]
      tunnel: w202 -> [w250 w288 w328 w436 w532 w604 w698 w786 w867 w911 w958 w1002 w1041 _ w1103 w1152 w1201 w1285 w1351 w1392 w1454 w1515 w1615 w1697 w1755 w1823]
      tunnel: w201 -> [w249 w287 w327 w435 w531 w603 w701 w789 w866 w910 w957 w1001 _ w1072 w1102 w1153 w1202 w1286 w1352 w1393 w1455 w1516 w1616 w1698 w1756 w1824]
      tunnel: [w252 w290 w330 w438 w534 w606 w700 w788 w869 w913 w952 w996 w1036 w1067 w1105 w1150 w1199 w1283 w1349 w1390 w1452 w1513 w1613 w1695 w1753 w1821] -> w200
      tunnel: [w251 w289 w329 w437 w533 w605 w699 w787 w868 w912 w959 w988 w1027 w1073 w1104 w1151 w1200 w1284 w1350 w1391 w1453 w1514 w1614 w1696 w1754 w1822] -> w199
      tunnel: [w250 w288 w328 w436 w532 w604 w698 w786 w867 w911 w958 w1002 w1041 w1066 w1103 w1152 w1201 w1285 w1351 w1392 w1454 w1515 w1615 w1697 w1755 w1823] -> w198
      tunnel: [w249 w287 w327 w435 w531 w603 w701 w789 w866 w910 w957 w1001 w1028 w1072 w1102 w1153 w1202 w1286 w1352 w1393 w1455 w1516 w1616 w1698 w1756 w1824] -> w197
      tunnel: w196 -> [_ _ _ w430 w528 _ w694 _ _ _ _ _ _ _ _ _ _ _ _ _ _ _ _ _ _ _]
      tunnel: w195 -> [_ _ _ w428 w527 _ _ _ _ _ _ _ _ _ _ _ _ _ _ _ _ _ _ _ _ _]
      tunnel: [w248 w283 w320 w356 w504 w593 w691 w775 w861 w904 w951 w987 w1026 w1065 w1101 w1134 w1191 w1248 w1343 w1379 w1445 w1507 w1567 w1653 w1745 w1814] -> w60
      tunnel: w194 -> [w248 w283 w320 w425 w504 w593 w691 w775 w861 w904 w951 w987 w1026 w1065 w1101 w1134 w1191 w1248 w1343 w1379 w1445 w1507 w1567 w1653 w1745 w1814]
      tunnel: w159 -> [_ _ _ w422 w501 w591 w688 w772 _ _ _ _ _ _ _ w1132 w1189 w1265 _ w1376 w1442 w1504 w1564 w1649 _ _]
      tunnel: w192 -> [_ _ _ w419 w500 w589 w687 w771 _ _ _ _ _ _ _ w1130 w1187 w1264 _ w1375 w1441 w1503 w1563 w1650 _ w1782]
      tunnel: w122 -> [_ _ _ w414 _ _ _ _ _ _ _ _ _ _ _ _ _ _ _ _ _ _ _ _ _ w1785]
      tunnel: [w247 w282 w319 w364 w503 w592 w690 w774 w860 w903 w950 w986 w1025 w1064 w1100 w1133 w1190 w1267 w1342 w1378 w1444 w1506 w1566 w1652 w1751 w1794] -> w124
      tunnel: w190 -> [w247 w282 w319 w418 w503 w592 w690 w774 w860 w903 w950 w986 w1025 w1064 w1100 w1133 w1190 w1267 w1342 w1378 w1444 w1506 w1566 w1652 w1751 w1794]
      tunnel: [w246 w281 w318 w355 w499 w588 w686 w770 w859 w902 w949 w985 w1024 w1063 w1099 w1129 w1186 w1247 w1341 w1374 w1440 w1502 w1562 w1648 w1740 w1810] -> w59
      tunnel: w164 -> [w246 w281 w318 w412 w499 w588 w686 w770 w859 w902 w949 w985 w1024 w1063 w1099 w1129 w1186 w1247 w1341 w1374 w1440 w1502 w1562 w1648 w1740 w1810]
      tunnel: [w245 w280 w317 w405 w498 w587 w676 w769 w858 w901 w948 w984 w1023 w1062 w1098 w1128 w1185 w1263 w1340 w1373 w1439 w1501 w1561 w1647 w1739 w1809] -> w92
      tunnel: w150 -> [w245 w280 w317 w405 w498 w587 w676 w769 w858 w901 w948 w984 w1023 w1062 w1098 w1128 w1185 w1263 w1340 w1373 w1439 w1501 w1561 w1647 w1738 w1783]
      tunnel: [w244 w279 w316 w404 w497 w586 w675 w768 w857 w900 w947 w983 w1022 w1061 w1097 w1127 w1184 w1262 w1339 w1372 w1438 w1500 w1560 w1646 w1724 w1796] -> w125
      tunnel: w143 -> [w244 w279 w316 w404 w497 w586 w675 w768 w857 w900 w947 w983 w1022 w1061 w1097 w1127 w1184 w1262 w1339 w1372 w1438 w1500 w1560 w1646 w1724 w1795]
      tunnel: [w243 w278 w315 w403 w496 w585 w674 w767 w856 w899 w946 w982 w1021 w1060 w1096 w1126 w1183 w1261 w1338 w1371 w1437 w1499 w1559 w1645 w1723 w1778] -> w104
      tunnel: w142 -> [w243 w278 w315 w403 w496 w585 w674 w767 w856 w899 w946 w982 w1021 w1060 w1096 w1126 w1183 w1261 w1338 w1371 w1437 w1499 w1559 w1645 w1723 w1776]
      tunnel: [w242 w277 w314 w402 w495 w584 w673 w766 w855 w898 w945 w981 w1020 w1059 w1095 w1125 w1182 w1260 w1337 w1370 w1436 w1498 w1558 w1644 w1722 w1775] -> w141
      tunnel: w140 -> [w242 w277 w314 w402 w495 w584 w673 w766 w855 w898 w945 w981 w1020 w1059 w1095 w1125 w1182 w1260 w1337 w1370 w1436 w1498 w1558 w1644 w1722 w1786]
      tunnel: w122 -> [_ _ _ _ _ _ _ _ _ _ _ _ _ _ _ _ _ _ _ _ _ _ _ _ _ w1774]
      tunnel: w121 -> [w241 w276 w313 w401 w494 w583 w672 w765 w854 w897 w944 w980 w1019 w1058 w1094 w1124 w1181 w1259 w1336 w1369 w1435 w1497 w1557 w1643 w1721 w1773]
      tunnel: [w241 w276 w313 w401 w494 w583 w672 w765 w854 w897 w944 w980 w1019 w1058 w1094 w1124 w1181 w1259 w1336 w1369 w1435 w1497 w1557 w1643 w1721 w1772] -> w97
      tunnel: [w240 w275 w312 w400 w493 w582 w671 w764 w853 w896 w943 w979 w1018 w1057 w1093 w1123 w1180 w1258 w1335 w1368 w1434 w1496 w1556 w1642 w1720 w1771] -> w96
      tunnel: w103 -> [w240 w275 w312 w400 w493 w582 w671 w764 w853 w896 w943 w979 w1018 w1057 w1093 w1123 w1180 w1258 w1335 w1368 w1434 w1496 w1556 w1642 w1720 w1770]
      tunnel: [w239 w274 w311 w399 w492 w581 w670 w763 w852 w895 w942 w978 w1017 w1056 w1092 w1122 w1179 w1257 w1334 w1367 w1433 w1495 w1555 w1641 w1719 w1768] -> w93
      tunnel: w95 -> [w239 w274 w311 w399 w492 w581 w670 w763 w852 w895 w942 w978 w1017 w1056 w1092 w1122 w1179 w1257 w1334 w1367 w1433 w1495 w1555 w1641 w1719 w1767]
      tunnel: [w237 w272 w309 w349 w489 w579 w668 w761 w850 w894 w941 w976 w1015 w1054 w1090 w1120 w1178 w1256 w1333 w1366 w1432 w1493 w1554 w1640 w1718 w1766] -> w53
      tunnel: w81 -> [w237 w272 w309 w395 w489 w579 w668 w761 w850 w894 w941 w976 w1015 w1054 w1090 w1120 w1178 w1256 w1333 w1366 w1432 w1493 w1554 w1640 w1718 w1766]
      tunnel: [w238 w273 w310 w350 w490 w580 w669 w762 w851 w893 w940 w977 w1016 w1055 w1091 w1121 w1177 w1255 w1332 w1365 w1431 w1494 w1553 w1639 w1717 w1765] -> w54
      tunnel: w80 -> [w238 w273 w310 w394 w490 w580 w669 w762 w851 w893 w940 w977 w1016 w1055 w1091 w1121 w1177 w1255 w1332 w1365 w1431 w1494 w1553 w1639 w1717 w1765]
      tunnel: [w230 w265 w302 w354 w486 w577 w666 w759 w843 w891 w938 w974 w1013 w1052 w1088 w1113 w1170 w1246 w1331 w1358 w1424 w1486 w1546 w1634 w1710 w1764] -> w58
      tunnel: w69 -> [w230 w265 w302 w384 w486 w577 w666 w759 w843 w891 w938 w974 w1013 w1052 w1088 w1113 w1170 w1246 w1331 w1358 w1424 w1486 w1546 w1634 w1710 w1764]
      tunnel: [w229 w264 w301 w353 w487 w578 w667 w760 w842 w892 w939 w975 w1014 w1053 w1089 w1112 w1169 w1245 w1330 w1357 w1423 w1485 w1545 w1633 w1709 w1763] -> w57
      tunnel: w68 -> [w229 w264 w301 w383 w487 w578 w667 w760 w842 w892 w939 w975 w1014 w1053 w1089 w1112 w1169 w1245 w1330 w1357 w1423 w1485 w1545 w1633 w1709 w1763]
      tunnel: [w232 w267 w304 w359 w485 w575 w664 w757 w848 w889 w936 w972 w1011 w1050 w1086 w1115 w1172 w1250 w1325 w1360 w1426 w1488 w1548 w1632 w1714 w1761] -> w51
      tunnel: w67 -> [w232 w267 w304 w380 w485 w575 w664 w757 w848 w889 w936 w972 w1011 w1050 w1086 w1115 w1172 w1250 w1325 w1360 w1426 w1488 w1548 w1632 w1714 w1761]
      tunnel: [w231 w266 w303 w357 w488 w576 w665 w758 w849 w890 w937 w973 w1012 w1051 w1087 w1114 w1171 w1249 w1324 w1359 w1425 w1487 w1547 w1631 w1713 w1762] -> w61
      tunnel: w66 -> [w231 w266 w303 w379 w488 w576 w665 w758 w849 w890 w937 w973 w1012 w1051 w1087 w1114 w1171 w1249 w1324 w1359 w1425 w1487 w1547 w1631 w1713 w1762]
      tunnel: [w234 w269 w306 w348 w484 w573 w662 w755 w846 w887 w934 w970 w1009 w1048 w1084 w1117 w1174 w1252 w1327 w1362 w1428 w1490 w1550 w1636 w1716 w1759] -> w52
      tunnel: w65 -> [w234 w269 w306 w376 w484 w573 w662 w755 w846 w887 w934 w970 w1009 w1048 w1084 w1117 w1174 w1252 w1327 w1362 w1428 w1490 w1550 w1636 w1716 w1759]
      tunnel: [w233 w268 w305 w347 w483 w574 w663 w756 w847 w888 w935 w971 w1010 w1049 w1085 w1116 w1173 w1251 w1326 w1361 w1427 w1489 w1549 w1635 w1715 w1760] -> w50
      tunnel: w64 -> [w233 w268 w305 w375 w483 w574 w663 w756 w847 w888 w935 w971 w1010 w1049 w1085 w1116 w1173 w1251 w1326 w1361 w1427 w1489 w1549 w1635 w1715 w1760]
      tunnel: [w236 w271 w308 w352 w482 w571 w660 w753 w844 w885 w932 w968 w1007 w1046 w1082 w1119 w1176 w1254 w1329 w1364 w1430 w1492 w1552 w1638 w1712 w1757] -> w56
      tunnel: w63 -> [w236 w271 w308 w372 w482 w571 w660 w753 w844 w885 w932 w968 w1007 w1046 w1082 w1119 w1176 w1254 w1329 w1364 w1430 w1492 w1552 w1638 w1712 w1757]
      tunnel: [w235 w270 w307 w351 w481 w572 w661 w754 w845 w886 w933 w969 w1008 w1047 w1083 w1118 w1175 w1253 w1328 w1363 w1429 w1491 w1551 w1637 w1711 w1758] -> w55
      tunnel: w62 -> [w235 w270 w307 w371 w481 w572 w661 w754 w845 w886 w933 w969 w1008 w1047 w1083 w1118 w1175 w1253 w1328 w1363 w1429 w1491 w1551 w1637 w1711 w1758]
      frame "wait" {
        n29 = Index Array(array=w263, index=0 ("Index")) -> (element=w261:string)
        n30 = Decimal String To Number(string=w261, default (0L)=u32 0) -> (number=w260:u32)  [unwired: 1 in, 1 out]
        n31 = Wait (ms)(milliseconds to wait=w260) -> ()  [unwired: 1 out]
      }
      frame "wait-min" {
        n32 = Index Array(array=w300, index=0 ("Index")) -> (element=w298:string)
        n33 = Decimal String To Number(string=w298, default (0L)=u32 0) -> (number=w286:u32)  [unwired: 1 in, 1 out]
        n34 = Multiply(x=w286, y=u32 60000) -> (x*y=w285:u32)
        n35 = Wait (ms)(milliseconds to wait=w285) -> ()  [unwired: 1 out]
      }
      frame "standby" {
        n36 = Index Array(array=w336, index=0 ("Index")) -> (element=w326:string)
        n37 = case shown="\"off\", Default" w326 {
          tunnel: [":PAGE:SCON:STAN 0" ":PAGE:SCON:STAN 1"] -> w321
          frame "off", Default {
          }
          frame "on" {
          }
        }
        n38 = VISA Write(VISA resource name=w325, write buffer=w321, error in (no error)=w324) -> (VISA resource name out=w323:refnum<visa-resource-name>, error out=w322:errorcluster)  [unwired: 1 out]
      }
      frame "transfer" {
        # "Adjusts graph colors."
        # "Adjusts graph colors."
        # "Is off"
        # "Is on"
        # "Ion will be the middle element of the array. The calculation of the index is done only once, since Is, Id, and Ig have the same dimensions."
        # "Ig off"
        # "Ig on"
        # "Is min"
        # "Is max"
        # "Ig min"
        # "Ig max"
        # "abs(Ig)"
        # "abs(Is)"
        # "Id min"
        # "Id max"
        # "Y1: Is\nY2: Id\nY3: Ig"
        # "abs(Id)"
        # "Adjusts graph colors."
        # "Adjusts graph colors."
        # "Id off"
        # "Id on"
        # "Don't connect the error lines\nof the two Split blocks!"
        # "Adjusts graph colors."
        # "Time array"
        n39 = Delete From Array(array=w467, index=0 ("Index")) -> (deleted portion=w465:string, array with subset deleted=w464:string[])  [unwired: 1 in]
        n40 = Bundle By Name(cluster=w428, "Emergency Stop"=w477) -> (w429:T2)
        n41 = Number To Decimal String(number=w422) -> (decimal integer string=w421:string)  [unwired: 1 in]
        n42 = case shown="\"d\", Default" w465 {
          tunnel: [w479 w480] -> w463
          frame "s" {
            w479 = u16 0 items=["Single", "Double"] ("sweep mode")
          }
          frame "d", Default {
            w480 = u16 1 items=["Single", "Double"] ("sweep mode")
          }
        }
        n43 = Fract/Exp String To Number(string=w464) -> (number=w449:dbl[])  [unwired: 3 in, 1 out]
        n44 = Concatenate Strings(w474, "Prefix (transfer)", w421, w419, "Suffix (transfer)") -> (w476:string)
        n45 = VISA Write(VISA resource name=w445, write buffer=":PAGE:CHAN:MODE SWE;" ("write buffer (\"\")"), error in (no error)=w444) -> (VISA resource name out=w442:refnum<visa-resource-name>, error out=w443:errorcluster)  [unwired: 1 out]
        n46 = String To Path(string=w476) -> (path=w473:path)
        n47 = Index Array(array=w449, index #1=0 ("Index")) -> (element #1=w462:dbl, element #2=w461:dbl, element #3=w460:dbl)  [unwired: 2 in]
        n48 = Delete From Array(array=w449, length=3 ("Length"), index=0 ("Index")) -> (array with subset deleted=w447:dbl[])  [unwired: 1 out]
        n49 = Build Array (concatenate)(w418, w414) -> (w364:i32[])
        n50 = Bundle By Name(cluster=w454, "Gate Start"=w462, "Gate Stop"=w461, "Gate Step (linear only)"=w460, "Gate Compliance"=w471, "Range mode"=w438, "Range"=w437) -> (w439:T4)
        n51 = control-ref of="Imax vs time"() -> (w393:refnum<vi>)
        n52 = control-ref of="Imin vs time"() -> (w392:refnum<vi>)
        n53 = control-ref of="Ion vs time"() -> (w361:refnum<vi>)
        n54 = control-ref of="Ioff vs time"() -> (w360:refnum<vi>)
        n55 = control-ref of="I vs Vg"() -> (w423:refnum<vi>)
        n56 = Index Array(array=w447, index #1=0 ("Index")) -> (element #1=w457:dbl, element #2=w456:dbl, element #3=w455:dbl)  [unwired: 2 in]
        n57 = call <vilib>:"compatOverwrite.vi"("overwrite (F)"=TRUE) -> ("overwrite?"=w427:T7)
        n58 = Bundle By Name(cluster=w453, "Drain Start"=w457, "Drain Stop"=w456, "Drain Step"=w455, "Drain Compliance"=w472, "Range mode"=w436, "Range"=w435) -> (w440:T5)
        n59 = call "4155C Transfer.vi"("VISA resource name in"=w442, "Gate"=w439, "Drain"=w440, "Timings"=w470, "error in (no error)"=w443, "SMU4"=w430, "sweep mode"=w463, "Panel Controls"=w429) -> ("VG"=w426:dbl[], "Outparams"=w434:T8, "VISA Resource Name out"=w469:refnum<visa-resource-name>, "IS"=w389:dbl[], "ID"=w391:dbl[], "IG"=w388:dbl[], "error out"=w415:errorcluster, "SMU4"=w431:dbl[])  [unwired: 12 in]
        n60 = Unbundle By Name(w434) -> ("V2 Step"=w433:dbl, "V2 Start"=w432:dbl, "Number of points"=w358:i32)
        n61 = Absolute Value(x=w389) -> (abs(x)=w374:dbl[])
        n62 = Absolute Value(x=w391) -> (abs(x)=w390:dbl[])
        n63 = Absolute Value(x=w388) -> (abs(x)=w377:dbl[])
        n64 = Array Size(array=w390) -> (size(s)=w398:i32)
        n65 = Divide(x=w398, y=2) -> (x/y=w341:dbl)
        n66 = Subtract(x=w341, y=1) -> (x-y=w340:dbl)
        n67 = Array Max & Min(array=w374) -> (max value=w381:dbl, min value=w382:dbl)  [unwired: 2 out]
        n68 = Array Max & Min(array=w390) -> (max value=w424:dbl, min value=w387:dbl)  [unwired: 2 out]
        n69 = Array Max & Min(array=w377) -> (max value=w386:dbl, min value=w385:dbl)  [unwired: 2 out]
        n70 = call "4155C Split array.vi"("Number of VAR2 steps"=w358, "Y2 data in"=w391, "X data in"=w426, "Y1 data in"=w389, "Y3 data in"=w388, "error in (no error)"=w415) -> ("Array of clusters"=w417:cluster{"Y data in":dbl[], "X data in":dbl[]}[], "error out"=w346:errorcluster)  [unwired: 1 in]
        n71 = Index Array(array=w374, index=w340) -> (element=w365:dbl)
        n72 = Index Array(array=w374, index=0) -> (element=w366:dbl)
        n73 = Index Array(array=w390, index=w340) -> (element=w367:dbl)
        n74 = Index Array(array=w390, index=0) -> (element=w368:dbl)
        n75 = Index Array(array=w377, index=w340) -> (element=w370:dbl)
        n76 = Index Array(array=w377, index=0) -> (element=w369:dbl)
        n77 = local write "Ig max"(w386) -> ()
        n78 = local write "Ig min"(w385) -> ()
        n79 = local write "Is max"(w381) -> ()
        n80 = local write "Is min"(w382) -> ()
        n81 = local write "Id max"(w424) -> ()
        n82 = local write "Id min"(w387) -> ()
        n83 = local write "I vs Vg"(w417) -> ()
        n84 = Build Array (concatenate)(w380, w381) -> (w359:dbl[])
        n85 = Build Array (concatenate)(w379, w382) -> (w357:dbl[])
        n86 = local write "Is off"(w366) -> ()
        n87 = local write "Is on"(w365) -> ()
        n88 = Build Array (concatenate)(w425, w424) -> (w356:dbl[])
        n89 = Build Array (concatenate)(w412, w387) -> (w355:dbl[])
        n90 = Build Array (concatenate)(w384, w386) -> (w354:dbl[])
        n91 = Build Array (concatenate)(w383, w385) -> (w353:dbl[])
        n92 = Build Array (concatenate)(w372, w365) -> (w352:dbl[])
        n93 = Build Array (concatenate)(w371, w366) -> (w351:dbl[])
        n94 = Build Array (concatenate)(w394, w367) -> (w350:dbl[])
        n95 = Build Array (concatenate)(w395, w368) -> (w349:dbl[])
        n96 = Build Array (concatenate)(w376, w370) -> (w348:dbl[])
        n97 = Build Array (concatenate)(w375, w369) -> (w347:dbl[])
        n98 = local write "Ig off"(w369) -> ()
        n99 = local write "Ig on"(w370) -> ()
        n100 = local write "Id off"(w368) -> ()
        n101 = local write "Id on"(w367) -> ()
        n102 = call "4155C Split array.vi"("Number of VAR2 steps"=w358, "Y2 data in"=w350, "X data in"=w364, "Y1 data in"=w352, "Y3 data in"=w348, "error in (no error)"=w346) -> ("Array of clusters"=w362:cluster{"Y data in":dbl[], "X data in":dbl[]}[], "error out"=w345:errorcluster)  [unwired: 1 in]
        n103 = call "4155C Split array.vi"("Number of VAR2 steps"=w358, "Y2 data in"=w349, "X data in"=w364, "Y1 data in"=w351, "Y3 data in"=w347, "error in (no error)"=w345) -> ("Array of clusters"=w363:cluster{"Y data in":dbl[], "X data in":dbl[]}[], "error out"=w344:errorcluster)  [unwired: 1 in]
        n104 = call "4155C Split array.vi"("Number of VAR2 steps"=w358, "Y2 data in"=w356, "X data in"=w364, "Y1 data in"=w359, "Y3 data in"=w354, "error in (no error)"=w344) -> ("Array of clusters"=w416:cluster{"Y data in":dbl[], "X data in":dbl[]}[], "error out"=w343:errorcluster)  [unwired: 1 in]
        n105 = call "4155C Split array.vi"("Number of VAR2 steps"=w358, "Y2 data in"=w355, "X data in"=w364, "Y1 data in"=w357, "Y3 data in"=w353, "error in (no error)"=w343) -> ("Array of clusters"=w413:cluster{"Y data in":dbl[], "X data in":dbl[]}[], "error out"=w342:errorcluster)  [unwired: 1 in]
        n106 = Open/Create/Replace File(file path (use dialog)=w473, error in=w342, operation (0:open)=w427) -> (refnum out=w410:refnum<file>, error out=w408:errorcluster)  [unwired: 3 in, 1 out]
        n107 = call "4155C Make Big 2d array.vi"("1D Var1"=w426, "1d IS"=w389, "1d ID"=w391, "1d IG"=w388, "1d SMU4"=w431, "SMU4"=w430, "VAR2 START"=w432, "Number of VAR2 steps"=w358, "VAR2 STEP"=w433, "VAR1 Name"="Vg", "Decimal places in header"=i8 1, "VAR2 Name"="Vd") -> ("Header array"=w411:string[], "Data array"=w409:dbl[][])  [unwired: 14 in]
        n108 = local write "Imax vs time"(w416) -> ()
        n109 = local write "Imin vs time"(w413) -> ()
        n110 = local write "Ion vs time"(w362) -> ()
        n111 = local write "Ioff vs time"(w363) -> ()
        n112 = call "4155C Config Chart Colours.vi"("Numeric"=w358, "XY Graph 2"=w393) -> ()  [unwired: 6 in]
        n113 = call "4155C Config Chart Colours.vi"("Numeric"=w358, "XY Graph 2"=w392) -> ()  [unwired: 6 in]
        n114 = call "4155C Config Chart Colours.vi"("Numeric"=w358, "XY Graph 2"=w361) -> ()  [unwired: 6 in]
        n115 = call "4155C Config Chart Colours.vi"("Numeric"=w358, "XY Graph 2"=w360) -> ()  [unwired: 6 in]
        n116 = call "4155C Config Chart Colours.vi"("Numeric"=w358, "XY Graph 2"=w423) -> ()  [unwired: 6 in]
        n117 = call "4155C Write array to file.vi"("Byte Stream File Refnum"=w410, "Header"=w411, "Data Array"=w409, "error in (no error)"=w408) -> ("dup refnum"=w407:refnum<file>, "error out"=w406:errorcluster)  [unwired: 1 in]
        n118 = Close File(refnum=w407, error in=w406) -> (error out=w468:errorcluster)  [unwired: 1 out]
      }
      frame "pulsedstressV" {
        w510 = 0
        n119 = Number To Decimal String(number=w501) -> (decimal integer string=w557:string)  [unwired: 1 in]
        n120 = Delete From Array(array=w491, index=0 ("Index")) -> (deleted portion=w548:string, array with subset deleted=w547:string[])  [unwired: 1 in]
        n121 = Bundle By Name(cluster=w527, "Emergency Stop"=w560) -> (w529:T2)
        n122 = VISA Write(VISA resource name=w541, write buffer=":PAGE:CHAN:MODE SWE;" ("write buffer (\"\")"), error in (no error)=w540) -> (VISA resource name out=w538:refnum<visa-resource-name>, error out=w539:errorcluster)  [unwired: 1 out]
        n123 = Concatenate Strings(w556, "-pulsedstressV-" ("Substring"), w557, w500, ".txt" ("Substring")) -> (w559:string)
        n124 = case shown="\"d\", Default" w548 {
          tunnel: [w569 w570] -> w546
          frame "s" {
            w569 = u16 0 items=["Single", "Double"] ("sweep mode")
          }
          frame "d", Default {
            w570 = u16 1 items=["Single", "Double"] ("sweep mode")
          }
        }
        n125 = Fract/Exp String To Number(string=w547) -> (number=w542:dbl[])  [unwired: 3 in, 1 out]
        n126 = String To Path(string=w559) -> (path=w555:path)
        n127 = Index Array(array=w542, index #1=0 ("Index")) -> (element #1=w519:dbl, element #2=w518:dbl, element #3=w515:dbl, element #4=w514:dbl, element #5=w513:dbl, element #6=w517:dbl)  [unwired: 5 in]
        n128 = Bundle By Name(cluster=w516, "Pulse period"=w514, "Base voltage"=w515, "Pulse width"=w513) -> (w512:T6)
        n129 = Unbundle By Name(w512) -> ("Pulse period"=w520:dbl)
        n130 = Bundle By Name(cluster=w544, "Gate Start"=w518, "Gate Stop"=w519, "Gate Step (linear only)"=0, "Gate Compliance"=w553, "Range mode"=w534, "Range"=w533) -> (w535:T4)
        n131 = call <vilib>:"compatOverwrite.vi"("overwrite (F)"=TRUE) -> ("overwrite?"=w505:T7)
        n132 = Bundle By Name(cluster=w543, "Drain Start"=w517, "Drain Stop"=w510, "Drain Step"=w510, "Drain Compliance"=w554, "Range mode"=w532, "Range"=w531) -> (w536:T5)
        n133 = call "4155C PulsedStressV.vi"("VISA resource name in"=w538, "sweep mode"=w546, "Panel Controls"=w529, "Gate"=w535, "Drain"=w536, "Timings"=w512, "error in (no error)"=w539, "SMU4"=w528) -> ("VISA Resource Name out"=w551:refnum<visa-resource-name>, "ID"=w508:dbl[], "IG"=w506:dbl[], "Outparams"=w530:T8, "error out"=w552:errorcluster)  [unwired: 3 in]
        n134 = Unbundle By Name(w530) -> ("Number of points"=w507:i32)  [unwired: 2 out]
        n135 = for {
          N: w507 -> [_]
          tunnel: [w566] -> w509 mode=indexing
          tunnel: w520 -> [w568]
          i -> [w567]
          n136 = Multiply(x=w568, y=w567) -> (x*y=w566:dbl)
        }
        n137 = Insert Into Array(array=dbl[][] [] ("Input Array"), new element=w509) -> (w521:dbl[][])  [unwired: 2 in]
        n138 = Insert Into Array(array=w521, new element=w508) -> (w526:dbl[][])  [unwired: 2 in]
        n139 = Insert Into Array(array=w526, new element=w506) -> (w525:dbl[][])  [unwired: 2 in]
        n140 = Transpose 2D Array(2D array=w525) -> (transposed array=w524:dbl[][])
        n141 = Open/Create/Replace File(file path (use dialog)=w555, error in=w552, operation (0:open)=w505) -> (refnum out=w563:refnum<file>, error out=w564:errorcluster)  [unwired: 3 in, 1 out]
        n142 = call "4155C Write array to file.vi"("Byte Stream File Refnum"=w563, "Header"=string[] ["Time /s", "Id /A", "Ig /A"], "Data Array"=w524, "error in (no error)"=w564) -> ("dup refnum"=w561:refnum<file>, "error out"=w562:errorcluster)  [unwired: 1 in]
        n143 = Close File(refnum=w561, error in=w562) -> (error out=w550:errorcluster)  [unwired: 1 out]
      }
      frame "transfer-fpp" {
        n144 = Number To Decimal String(number=w591) -> (decimal integer string=w645:string)  [unwired: 1 in]
        n145 = Bundle By Name(cluster=w621, "Emergency Stop"=w649) -> (w657:T1)
        n146 = Delete From Array(array=w636, index=0 ("Index")) -> (deleted portion=w634:string, array with subset deleted=w633:string[])  [unwired: 1 in]
        n147 = Concatenate Strings(w644, "-transferfpp-" ("Substring"), w645, w589, ".txt" ("Substring")) -> (w647:string)
        n148 = VISA Write(VISA resource name=w613, write buffer=":PAGE:CHAN:MODE SWE;" ("write buffer (\"\")"), error in (no error)=w612) -> (VISA resource name out=w610:refnum<visa-resource-name>, error out=w611:errorcluster)  [unwired: 1 out]
        n149 = case shown="\"d\", Default" w634 {
          tunnel: [w658 w659] -> w632
          frame "s" {
            w658 = u16 0 items=["Single", "Double"] ("sweep mode")
          }
          frame "d", Default {
            w659 = u16 1 items=["Single", "Double"] ("sweep mode")
          }
        }
        n150 = Fract/Exp String To Number(string=w633) -> (number=w617:dbl[])  [unwired: 3 in, 1 out]
        n151 = String To Path(string=w647) -> (path=w643:path)
        n152 = Index Array(array=w617, index #1=0 ("Index")) -> (element #1=w631:dbl, element #2=w630:dbl, element #3=w629:dbl)  [unwired: 2 in]
        n153 = Delete From Array(array=w617, length=3 ("Length"), index=0 ("Index")) -> (array with subset deleted=w615:dbl[])  [unwired: 1 out]
        n154 = Bundle By Name(cluster=w623, "Gate Start"=w631, "Gate Stop"=w630, "Gate Step (linear only)"=w629, "Gate Compliance"=w641, "Range mode"=w606, "Range"=w605) -> (w607:T4)
        n155 = Index Array(array=w615, index #1=0 ("Index")) -> (element #1=w626:dbl, element #2=w625:dbl, element #3=w624:dbl)  [unwired: 2 in]
        n156 = call <vilib>:"compatOverwrite.vi"("overwrite (F)"=TRUE) -> ("overwrite?"=w594:T7)
        n157 = Bundle By Name(cluster=w622, "Drain Start"=w626, "Drain Stop"=w625, "Drain Step"=w624, "Drain Compliance"=w642, "Range mode"=w604, "Range"=w603) -> (w608:T5)
        n158 = call "4155C Transfer-FPP.vi"("VISA resource name in"=w610, "Gate"=w607, "Drain"=w608, "Timings"=w640, "error in (no error)"=w611, "sweep mode"=w632, "Panel Controls"=w657) -> ("VG"=w648:dbl[], "Outparams"=w602:T8, "VISA Resource Name out"=w638:refnum<visa-resource-name>, "Vprobe2"=w598:dbl[], "ID"=w597:dbl[], "IG"=w596:dbl[], "Vprobe1"=w595:dbl[], "error out"=w639:errorcluster)  [unwired: 13 in]
        n159 = Unbundle By Name(w602) -> ("V2 Step"=w601:dbl, "V2 Start"=w600:dbl, "Number of points"=w599:i32)
        n160 = Open/Create/Replace File(file path (use dialog)=w643, error in=w639, operation (0:open)=w594) -> (refnum out=w654:refnum<file>, error out=w655:errorcluster)  [unwired: 3 in, 1 out]
        n161 = call "4155C Make Big 2d array FPP.vi"("1D Var1"=w648, "1d ID"=w597, "1d Vp2"=w598, "1d IG"=w596, "1d Vp1"=w595, "VAR2 START"=w600, "Number of VAR2 steps"=w599, "VAR2 STEP"=w601, "VAR1 Name"="Vg", "Decimal places in header"=i8 1, "VAR2 Name"="Vd") -> ("Header array"=w650:string[], "Data array"=w651:dbl[][])  [unwired: 15 in]
        n162 = call "4155C Write array to file.vi"("Byte Stream File Refnum"=w654, "Header"=w650, "Data Array"=w651, "error in (no error)"=w655) -> ("dup refnum"=w652:refnum<file>, "error out"=w653:errorcluster)  [unwired: 1 in]
        n163 = Close File(refnum=w652, error in=w653) -> (error out=w637:errorcluster)  [unwired: 1 out]
      }
      frame "output" {
        n164 = Number To Decimal String(number=w688) -> (decimal integer string=w737:string)  [unwired: 1 in]
        n165 = Bundle By Name(cluster=w714, "Emergency Stop"=w740) -> (w750:T1)
        n166 = Delete From Array(array=w729, index=0 ("Index")) -> (deleted portion=w727:string, array with subset deleted=w726:string[])  [unwired: 1 in]
        n167 = Concatenate Strings(w736, "Prefix (output)", w737, w687, "Suffix (output)") -> (w739:string)
        n168 = VISA Write(VISA resource name=w705, write buffer=":PAGE:CHAN:MODE SWE;" ("write buffer (\"\")"), error in (no error)=w702) -> (VISA resource name out=w704:refnum<visa-resource-name>, error out=w703:errorcluster)  [unwired: 1 out]
        n169 = case shown="\"d\", Default" w727 {
          tunnel: [w751 w752] -> w725
          frame "s" {
            w751 = u16 0 items=["Single", "Double"] ("sweep mode")
          }
          frame "d", Default {
            w752 = u16 1 items=["Single", "Double"] ("sweep mode")
          }
        }
        n170 = Fract/Exp String To Number(string=w726) -> (number=w708:dbl[])  [unwired: 3 in, 1 out]
        n171 = String To Path(string=w739) -> (path=w735:path)
        n172 = Index Array(array=w708, index #1=0 ("Index")) -> (element #1=w724:dbl, element #2=w723:dbl, element #3=w722:dbl)  [unwired: 2 in]
        n173 = Delete From Array(array=w708, length=3 ("Length"), index=0 ("Index")) -> (array with subset deleted=w707:dbl[])  [unwired: 1 out]
        n174 = control-ref of="I vs Vd"() -> (w678:refnum<vi>)
        n175 = Bundle By Name(cluster=w716, "Gate Start"=w724, "Gate Stop"=w723, "Gate Step (linear only)"=w722, "Gate Compliance"=w733, "Range mode"=w700, "Range"=w699) -> (w749:T4)
        n176 = Index Array(array=w707, index #1=0 ("Index")) -> (element #1=w719:dbl, element #2=w718:dbl, element #3=w717:dbl)  [unwired: 2 in]
        n177 = call <vilib>:"compatOverwrite.vi"("overwrite (F)"=TRUE) -> ("overwrite?"=w692:T7)
        n178 = Bundle By Name(cluster=w715, "Drain Start"=w719, "Drain Stop"=w718, "Drain Step"=w717, "Drain Compliance"=w734, "Range mode"=w698, "Range"=w701) -> (w748:T5)
        n179 = call "4155C Output.vi"("VISA resource name in"=w704, "Gate"=w749, "Drain"=w748, "Timings"=w732, "error in (no error)"=w703, "SMU4"=w694, "sweep mode"=w725, "Panel controls"=w750) -> ("VD"=w685:dbl[], "Outparams"=w696:T8, "VISA Resource Name out"=w731:refnum<visa-resource-name>, "IS"=w684:dbl[], "ID"=w683:dbl[], "IG"=w682:dbl[], "error out"=w680:errorcluster, "SMU4"=w693:dbl[])  [unwired: 12 in]
        n180 = Unbundle By Name(w696) -> ("V2 Step"=w697:dbl, "V2 Start"=w695:dbl, "Number of points"=w677:i32)
        n181 = call "4155C Split array.vi"("Number of VAR2 steps"=w677, "Y2 data in"=w683, "X data in"=w685, "Y1 data in"=w684, "Y3 data in"=w682, "error in (no error)"=w680) -> ("Array of clusters"=w681:cluster{"Y data in":dbl[], "X data in":dbl[]}[], "error out"=w679:errorcluster)  [unwired: 1 in]
        n182 = local write "I vs Vd"(w681) -> ()
        n183 = call "4155C Config Chart Colours.vi"("Numeric"=w677, "XY Graph 2"=w678) -> ()  [unwired: 6 in]
        n184 = Open/Create/Replace File(file path (use dialog)=w735, error in=w679, operation (0:open)=w692) -> (refnum out=w745:refnum<file>, error out=w746:errorcluster)  [unwired: 3 in, 1 out]
        n185 = call "4155C Make Big 2d array.vi"("1D Var1"=w685, "1d IS"=w684, "1d ID"=w683, "1d IG"=w682, "1d SMU4"=w693, "SMU4"=w694, "VAR2 START"=w695, "Number of VAR2 steps"=w677, "VAR2 STEP"=w697, "VAR1 Name"="Vd", "Decimal places in header"=i8 1, "VAR2 Name"="Vg") -> ("Header array"=w741:string[], "Data array"=w742:dbl[][])  [unwired: 14 in]
        n186 = call "4155C Write array to file.vi"("Byte Stream File Refnum"=w745, "Header"=w741, "Data Array"=w742, "error in (no error)"=w746) -> ("dup refnum"=w743:refnum<file>, "error out"=w744:errorcluster)  [unwired: 1 in]
        n187 = Close File(refnum=w743, error in=w744) -> (error out=w730:errorcluster)  [unwired: 1 out]
      }
      frame "output-fpp" {
        n188 = Number To Decimal String(number=w772) -> (decimal integer string=w826:string)  [unwired: 1 in]
        n189 = Bundle By Name(cluster=w802, "Emergency Stop"=w829) -> (w839:T1)
        n190 = Delete From Array(array=w817, index=0 ("Index")) -> (deleted portion=w815:string, array with subset deleted=w814:string[])  [unwired: 1 in]
        n191 = VISA Write(VISA resource name=w793, write buffer=":PAGE:CHAN:MODE SWE;" ("write buffer (\"\")"), error in (no error)=w790) -> (VISA resource name out=w792:refnum<visa-resource-name>, error out=w791:errorcluster)  [unwired: 1 out]
        n192 = Concatenate Strings(w825, "-outputfpp-" ("Substring"), w826, w771, ".txt" ("Substring")) -> (w828:string)
        n193 = case shown="\"d\", Default" w815 {
          tunnel: [w840 w841] -> w813
          frame "s" {
            w840 = u16 0 items=["Single", "Double"] ("sweep mode")
          }
          frame "d", Default {
            w841 = u16 1 items=["Single", "Double"] ("sweep mode")
          }
        }
        n194 = Fract/Exp String To Number(string=w814) -> (number=w796:dbl[])  [unwired: 3 in, 1 out]
        n195 = String To Path(string=w828) -> (path=w824:path)
        n196 = Index Array(array=w796, index #1=0 ("Index")) -> (element #1=w812:dbl, element #2=w811:dbl, element #3=w810:dbl)  [unwired: 2 in]
        n197 = Delete From Array(array=w796, length=3 ("Length"), index=0 ("Index")) -> (array with subset deleted=w795:dbl[])  [unwired: 1 out]
        n198 = Bundle By Name(cluster=w804, "Gate Start"=w812, "Gate Stop"=w811, "Gate Step (linear only)"=w810, "Gate Compliance"=w822, "Range mode"=w788, "Range"=w787) -> (w838:T4)
        n199 = Index Array(array=w795, index #1=0 ("Index")) -> (element #1=w807:dbl, element #2=w806:dbl, element #3=w805:dbl)  [unwired: 2 in]
        n200 = call <vilib>:"compatOverwrite.vi"("overwrite (F)"=TRUE) -> ("overwrite?"=w776:T7)
        n201 = Bundle By Name(cluster=w803, "Drain Start"=w807, "Drain Stop"=w806, "Drain Step"=w805, "Drain Compliance"=w823, "Range mode"=w786, "Range"=w789) -> (w837:T5)
        n202 = call "4155C Output-FPP.vi"("VISA resource name in"=w792, "Gate"=w838, "Drain"=w837, "Timings"=w821, "error in (no error)"=w791, "sweep mode"=w813, "Panel controls"=w839) -> ("VD"=w781:dbl[], "Outparams"=w784:T8, "VISA Resource Name out"=w819:refnum<visa-resource-name>, "Vprobe2"=w780:dbl[], "ID"=w779:dbl[], "IG"=w778:dbl[], "Vprobe1"=w777:dbl[], "error out"=w820:errorcluster)  [unwired: 13 in]
        n203 = Unbundle By Name(w784) -> ("V2 Step"=w785:dbl, "V2 Start"=w783:dbl, "Number of points"=w782:i32)
        n204 = Open/Create/Replace File(file path (use dialog)=w824, error in=w820, operation (0:open)=w776) -> (refnum out=w834:refnum<file>, error out=w835:errorcluster)  [unwired: 3 in, 1 out]
        n205 = call "4155C Make Big 2d array FPP.vi"("1D Var1"=w781, "1d ID"=w779, "1d Vp2"=w780, "1d IG"=w778, "1d Vp1"=w777, "VAR2 START"=w783, "Number of VAR2 steps"=w782, "VAR2 STEP"=w785, "VAR1 Name"="Vd", "Decimal places in header"=i8 1, "VAR2 Name"="Vg") -> ("Header array"=w830:string[], "Data array"=w831:dbl[][])  [unwired: 15 in]
        n206 = call "4155C Write array to file.vi"("Byte Stream File Refnum"=w834, "Header"=w830, "Data Array"=w831, "error in (no error)"=w835) -> ("dup refnum"=w832:refnum<file>, "error out"=w833:errorcluster)  [unwired: 1 in]
        n207 = Close File(refnum=w832, error in=w833) -> (error out=w818:errorcluster)  [unwired: 1 out]
      }
      frame "itime" {
        n208 = Delete From Array(array=w873, index=0 ("Index")) -> (deleted portion=w874:string)  [unwired: 1 in, 1 out]
        n209 = case shown="\"s\"" w874 {
          tunnel: w872 -> [w878 w880 w883]
          tunnel: [w877 w879 w882] -> w865
          frame "s" {
            w876 = u32 0 items=["short  ", "medium  ", "long  "] ("integration time 2")
            n210 = Bundle By Name(cluster=w878, "integration time"=w876) -> (w877:T6)
          }
          frame "m", Default {
            w881 = u32 1 items=["short  ", "medium  ", "long  "] ("integration time 2")
            n211 = Bundle By Name(cluster=w880, "integration time"=w881) -> (w879:T6)
          }
          frame "l" {
            w884 = u32 2 items=["short  ", "medium  ", "long  "] ("integration time 2")
            n212 = Bundle By Name(cluster=w883, "integration time"=w884) -> (w882:T6)
          }
        }
      }
      frame "pulsed" {
        n213 = Delete From Array(array=w917, index=0 ("Index")) -> (deleted portion=w918:string, array with subset deleted=w905:string[])  [unwired: 1 in]
        n214 = case shown="\"on\", Default" w918 {
          tunnel: w916 -> [w928 w931]
          tunnel: [w927 w930] -> w909
          tunnel: w905 -> [w925 _]
          frame "on", Default {
            w926 = u16 1 items=["Continuous", "Pulsed"] ("sweep method")
            n215 = Fract/Exp String To Number(string=w925) -> (number=w923:dbl[])  [unwired: 3 in, 1 out]
            n216 = Index Array(array=w923, index #1=0 ("Index")) -> (element #1=w922:dbl, element #2=w921:dbl, element #3=w920:dbl)  [unwired: 2 in]
            n217 = Bundle By Name(cluster=w928, "sweep method"=w926, "Pulse period"=w922, "Base voltage"=w921, "Pulse width"=w920) -> (w927:T6)
          }
          frame "off" {
            w929 = u16 0 items=["Continuous", "Pulsed"] ("sweep method")
            n218 = Bundle By Name(cluster=w931, "sweep method"=w929) -> (w930:T6)
          }
        }
      }
      frame "gaterangemode" {
        n219 = Delete From Array(array=w962, index=0 ("Index")) -> (deleted portion=w963:string)  [unwired: 1 in, 1 out]
        n220 = case shown="\"f\"" w963 {
          tunnel: [w965 w966 w967] -> w952
          frame "a", Default {
            w965 = u16 0 items=["Auto", "Limited", "Fixed"] ("Gate Range\nmode 2")
          }
          frame "f" {
            w966 = u16 2 items=["Auto", "Limited", "Fixed"] ("Gate Range\nmode 2")
          }
          frame "l" {
            w967 = u16 1 items=["Auto", "Limited", "Fixed"] ("Gate Range\nmode 2")
          }
        }
      }
      frame "gaterange" {
        (unwired) u8 11 items=["10fA  ", "100fA  ", "1nA  ", "10nA", "100nA", "1uA", "10uA", "100uA", "1mA", "10mA", "100mA", "1A"] ("Gate Range 2")
        n221 = Delete From Array(array=w1005, index=0 ("Index")) -> (deleted portion=w995:string)  [unwired: 1 in, 1 out]
        n222 = Scan Value(string=w995, format string="") -> (value=w993:dbl)  [unwired: 1 in, 1 out]
        n223 = Logarithm Base 10(1:w993) -> (0:w992:dbl)
        n224 = Round To Nearest(number=w992) -> (nearest integer value=w991:dbl)
        n225 = Add(x=w991, y=11.0) -> (x+y=w989:dbl)
        n226 = To Unsigned Byte Integer(number=w989) -> (unsigned 8bit integer=w988:u8)
      }
      frame "drainrange" {
        (unwired) u8 11 items=["10fA  ", "100fA  ", "1nA  ", "10nA", "100nA", "1uA", "10uA", "100uA", "1mA", "10mA", "100mA", "1A"] ("Gate Range 2")
        n227 = Delete From Array(array=w1044, index=0 ("Index")) -> (deleted portion=w1035:string)  [unwired: 1 in, 1 out]
        n228 = Scan Value(string=w1035, format string="") -> (value=w1033:dbl)  [unwired: 1 in, 1 out]
        n229 = Logarithm Base 10(1:w1033) -> (0:w1032:dbl)
        n230 = Round To Nearest(number=w1032) -> (nearest integer value=w1031:dbl)
        n231 = Add(x=w1031, y=11.0) -> (x+y=w1029:dbl)
        n232 = To Unsigned Byte Integer(number=w1029) -> (unsigned 8bit integer=w1028:u8)
      }
      frame "drainrangemode" {
        n233 = Delete From Array(array=w1076, index=0 ("Index")) -> (deleted portion=w1077:string)  [unwired: 1 in, 1 out]
        n234 = case shown="\"f\"" w1077 {
          tunnel: [w1079 w1080 w1081] -> w1066
          frame "a", Default {
            w1079 = u16 0 items=["Auto", "Limited", "Fixed"] ("Gate Range\nmode 2")
          }
          frame "f" {
            w1080 = u16 2 items=["Auto", "Limited", "Fixed"] ("Gate Range\nmode 2")
          }
          frame "l" {
            w1081 = u16 1 items=["Auto", "Limited", "Fixed"] ("Gate Range\nmode 2")
          }
        }
      }
      frame "Error", Default {
      }
      frame "logfile" {
        n235 = Number To Decimal String(number=w1132) -> (decimal integer string=w1167:string)  [unwired: 1 in]
        n236 = Concatenate Strings(w1166, "logfile" ("Substring"), w1167, w1130, ".txt" ("Substring")) -> (w1164:string)
        n237 = String To Path(string=w1164) -> (path=w1137:path)
        n238 = Unbundle(w1163) -> ("integration time"=w1162:u32, "Short/Long integration time"=w1161:dbl, "hold time (sec)"=w1160:dbl, "delay time (sec)"=w1159:dbl, "Step Time (0 disables)"=w1158:dbl, "sweep method"=w1157:u16, "Pulse period"=w1156:dbl, "Base voltage"=w1155:dbl, "Pulse width"=w1154:dbl)
        n239 = Build Array(w1162, w1161, w1160, w1159, w1158, w1157, w1156, w1155, w1154, w1148, w1149, w1150, w1151, w1152, w1153) -> (w1141:dbl[])
        n240 = Insert Into Array(array=dbl[][] [] ("Input Array"), new element=w1141) -> (w1140:dbl[][])  [unwired: 2 in]
        n241 = call <vilib>:"compatOverwrite.vi"("overwrite (F)"=TRUE) -> ("overwrite?"=w1135:T7)
        n242 = Open/Create/Replace File(file path (use dialog)=w1137, error in=w1139, operation (0:open)=w1135) -> (refnum out=w1145:refnum<file>, error out=w1144:errorcluster)  [unwired: 3 in, 1 out]
        n243 = call "4155C Write array to file.vi"("Byte Stream File Refnum"=w1145, "Header"=string[] ["Int Time", "Short/Long Itime", "Hold time", "Delay time", "Step time", "Sweep method", "Pulse period", "Base Voltage", "Pulse width", "Drain compliance", "Gate compliance", "Gate range mode", "Gate range", "S/D range mode", "S/D range"], "Data Array"=w1140, "error in (no error)"=w1144) -> ("dup refnum"=w1147:refnum<file>, "error out"=w1146:errorcluster)  [unwired: 1 in]
        n244 = Close File(refnum=w1147, error in=w1146) -> (error out=w1138:errorcluster)  [unwired: 1 out]
      }
      frame "sample" {
        n245 = Number To Decimal String(number=w1189) -> (decimal integer string=w1237:string)  [unwired: 1 in]
        n246 = Fract/Exp String To Number(string=w1234) -> (number=w1195:dbl[])  [unwired: 3 in, 1 out]
        n247 = Concatenate Strings(w1212, "-sample-" ("Substring"), w1237, w1187, ".txt" ("Substring")) -> (w1235:string)
        n248 = Index Array(array=w1195, index=0 ("Index")) -> (element=w1232:dbl)
        n249 = String To Path(string=w1235) -> (path=w1216:path)
        n250 = Index Array(array=w1195, index=2 ("Index")) -> (element=w1228:dbl)
        n251 = Index Array(array=w1195, index=3 ("Index")) -> (element=w1197:dbl)
        n252 = Index Array(array=w1195, index=4 ("Index")) -> (element=w1194:dbl)
        n253 = call "4155C Config Sampling Measurements.vi"("Sampling interval"=w1194, "Sample time"=w1197, "Display on/off"=TRUE, "Timings"=w1203, "Num Points"=w1228, "error in (no error)"=w1239, "Drain Compliance"=w1238, "Gate Compliance"=w1213, "VISA session"=w1240) -> ("error out"=w1241:errorcluster, "dup VISA resource name"=w1242:refnum<visa-resource-name>)  [unwired: 1 in]
        n254 = Index Array(array=w1195, index=1 ("Index")) -> (element=w1229:dbl)
        n255 = call "4155C Take Sample.vi"("Emergency Stop"=w1209, "error in (no error)"=w1241, "Vd"=w1229, "Vg"=w1232, "VISA resource name in"=w1242) -> ("error out"=w1207:errorcluster, "Id"=w1244:dbl[], "Ig"=w1218:dbl[], "VISA Resource Name out"=w1205:refnum<visa-resource-name>, "Is"=w1243:dbl[], "Time"=w1222:dbl[])  [unwired: 1 in]
        n256 = Insert Into Array(array=dbl[][] [] ("Input Array"), new element=w1222) -> (w1221:dbl[][])  [unwired: 2 in]
        n257 = Insert Into Array(array=w1221, new element=w1218) -> (w1220:dbl[][])  [unwired: 2 in]
        n258 = Insert Into Array(array=w1220, new element=w1244) -> (w1219:dbl[][])  [unwired: 2 in]
        n259 = VISA Write(VISA resource name=w1205, write buffer=":DISP ON" ("write buffer (\"\")"), error in (no error)=w1207) -> (VISA resource name out=w1204:refnum<visa-resource-name>, error out=w1206:errorcluster)  [unwired: 1 out]
        n260 = Insert Into Array(array=w1219, new element=w1243) -> (w1211:dbl[][])  [unwired: 2 in]
        n261 = Transpose 2D Array(2D array=w1211) -> (transposed array=w1210:dbl[][])
        n262 = call <vilib>:"compatOverwrite.vi"("overwrite (F)"=TRUE) -> ("overwrite?"=w1192:T7)
        n263 = Open/Create/Replace File(file path (use dialog)=w1216, error in=w1206, operation (0:open)=w1192) -> (refnum out=w1225:refnum<file>, error out=w1224:errorcluster)  [unwired: 3 in, 1 out]
        n264 = call "4155C Write array to file.vi"("Byte Stream File Refnum"=w1225, "Header"=string[] ["Time /s", "Ig /A", "Id /A", "Is /A"], "Data Array"=w1210, "error in (no error)"=w1224) -> ("dup refnum"=w1227:refnum<file>, "error out"=w1226:errorcluster)  [unwired: 1 in]
        n265 = Close File(refnum=w1227, error in=w1226) -> (error out=w1214:errorcluster)  [unwired: 1 out]
      }
      frame "samplei" {
        n266 = Number To Decimal String(number=w1265) -> (decimal integer string=w1316:string)  [unwired: 1 in]
        n267 = Concatenate Strings(w1295, "-samplei-" ("Substring"), w1316, w1264, ".txt" ("Substring")) -> (w1314:string)
        n268 = Fract/Exp String To Number(string=w1313) -> (number=w1280:dbl[])  [unwired: 3 in, 1 out]
        n269 = String To Path(string=w1314) -> (path=w1298:path)
        n270 = Index Array(array=w1280, index=4 ("Index")) -> (element=w1274:dbl)
        n271 = Index Array(array=w1280, index=3 ("Index")) -> (element=w1275:dbl)
        n272 = Index Array(array=w1280, index=1 ("Index")) -> (element=w1277:dbl)
        n273 = Index Array(array=w1280, index=0 ("Index")) -> (element=w1278:dbl)
        n274 = Index Array(array=w1280, index=2 ("Index")) -> (element=w1276:dbl)
        n275 = call "4155C Config SamplingI Measurements.vi"("Sample time"=w1276, "Display on/off"=TRUE, "Timings"=w1287, "Num Points"=w1277, "error in (no error)"=w1318, "Sampling interval"=w1275, "VISA session"=w1319) -> ("error out"=w1320:errorcluster, "dup VISA resource name"=w1321:refnum<visa-resource-name>)  [unwired: 3 in]
        n276 = call "4155C Take SampleI.vi"("Emergency Stop"=w1292, "error in (no error)"=w1320, "Idg 2"=w1278, "Vdg compliance 2"=w1274, "VISA resource name in"=w1321) -> ("error out"=w1290:errorcluster, "Idg"=w1323:dbl[], "Vdg"=w1300:dbl[], "VISA Resource Name out"=w1288:refnum<visa-resource-name>, "Is"=w1322:dbl[], "Time"=w1304:dbl[])  [unwired: 1 in]
        n277 = Insert Into Array(array=dbl[][] [] ("Input Array"), new element=w1304) -> (w1303:dbl[][])  [unwired: 2 in]
        n278 = Insert Into Array(array=w1303, new element=w1300) -> (w1302:dbl[][])  [unwired: 2 in]
        n279 = Insert Into Array(array=w1302, new element=w1323) -> (w1301:dbl[][])  [unwired: 2 in]
        n280 = VISA Write(VISA resource name=w1288, write buffer=":DISP ON" ("write buffer (\"\")"), error in (no error)=w1290) -> (VISA resource name out=w1273:refnum<visa-resource-name>, error out=w1289:errorcluster)  [unwired: 1 out]
        n281 = Insert Into Array(array=w1301, new element=w1322) -> (w1294:dbl[][])  [unwired: 2 in]
        n282 = call <vilib>:"compatOverwrite.vi"("overwrite (F)"=TRUE) -> ("overwrite?"=w1268:T7)
        n283 = Open/Create/Replace File(file path (use dialog)=w1298, error in=w1289, operation (0:open)=w1268) -> (refnum out=w1307:refnum<file>, error out=w1306:errorcluster)  [unwired: 3 in, 1 out]
        n284 = Transpose 2D Array(2D array=w1294) -> (transposed array=w1293:dbl[][])
        n285 = call "4155C Write array to file.vi"("Byte Stream File Refnum"=w1307, "Header"=string[] ["Time /s", "Vdg /V", "Idg /A", "Is /A"], "Data Array"=w1293, "error in (no error)"=w1306) -> ("dup refnum"=w1309:refnum<file>, "error out"=w1308:errorcluster)  [unwired: 1 in]
        n286 = Close File(refnum=w1309, error in=w1308) -> (error out=w1271:errorcluster)  [unwired: 1 out]
        n287 = VISA Write(VISA resource name=w1273, write buffer=";:PAGE:SCON:STAN OFF;:PAGE:CHAN:VSU2:DIS;" ("write buffer (\"\")"), error in (no error)=w1271) -> (VISA resource name out=w1269:refnum<visa-resource-name>, error out=w1270:errorcluster)  [unwired: 1 out]
      }
      frame "#" {
        n288 = VISA Write(VISA resource name=w1348, write buffer=":DISP ON" ("write buffer (\"\")"), error in (no error)=w1347) -> (VISA resource name out=w1346:refnum<visa-resource-name>, error out=w1345:errorcluster)  [unwired: 1 out]
      }
      frame "stressV" {
        n289 = Number To Decimal String(number=w1376) -> (decimal integer string=w1417:string)  [unwired: 1 in]
        n290 = Concatenate Strings(w1401, "-stressV-" ("Substring"), w1417, w1375, ".txt" ("Substring")) -> (w1415:string)
        n291 = Fract/Exp String To Number(string=w1414) -> (number=w1387:dbl[])  [unwired: 3 in, 1 out]
        n292 = String To Path(string=w1415) -> (path=w1405:path)
        n293 = Index Array(array=w1387, index=3 ("Index")) -> (element=w1384:dbl)
        n294 = Index Array(array=w1387, index=1 ("Index")) -> (element=w1382:dbl)
        n295 = Index Array(array=w1387, index=0 ("Index")) -> (element=w1381:dbl)
        n296 = Index Array(array=w1387, index=4 ("Index")) -> (element=w1386:dbl)
        n297 = Index Array(array=w1387, index=2 ("Index")) -> (element=w1383:dbl)
        n298 = call "4155C Config V Stress.vi"("VISA session"=w1420, "ID compliance"=w1384, "VD"=w1382, "VG"=w1381, "IG compliance"=w1383, "error in (no error)"=w1419, "Display on/off"=TRUE) -> ("dup VISA resource name"=w1422:refnum<visa-resource-name>, "error out"=w1421:errorcluster)
        n299 = call "4155C Apply Stress.vi"("error in (no error)"=w1421, "Duration"=w1386, "Emergency Stop"=w1400, "VISA resource name in"=w1422) -> ("error out"=w1398:errorcluster, "VISA Resource Name out"=w1396:refnum<visa-resource-name>)
        n300 = VISA Write(VISA resource name=w1396, write buffer=":DISP ON" ("write buffer (\"\")"), error in (no error)=w1398) -> (VISA resource name out=w1395:refnum<visa-resource-name>, error out=w1397:errorcluster)  [unwired: 1 out]
        n301 = call <vilib>:"compatOverwrite.vi"("overwrite (F)"=TRUE) -> ("overwrite?"=w1380:T7)
        n302 = Open/Create/Replace File(file path (use dialog)=w1405, error in=w1397, operation (0:open)=w1380) -> (refnum out=w1408:refnum<file>, error out=w1407:errorcluster)  [unwired: 3 in, 1 out]
        n303 = call "4155C Write array to file.vi"("Byte Stream File Refnum"=w1408, "Header"=string[] ["V stress completed successfully", ""], "error in (no error)"=w1407) -> ("dup refnum"=w1410:refnum<file>, "error out"=w1409:errorcluster)  [unwired: 2 in]
        n304 = Close File(refnum=w1410, error in=w1409) -> (error out=w1403:errorcluster)  [unwired: 1 out]
      }
      frame "stressI" {
        n305 = Number To Decimal String(number=w1442) -> (decimal integer string=w1479:string)  [unwired: 1 in]
        n306 = Concatenate Strings(w1463, "-stressI-" ("Substring"), w1479, w1441, ".txt" ("Substring")) -> (w1477:string)
        n307 = Fract/Exp String To Number(string=w1476) -> (number=w1451:dbl[])  [unwired: 3 in, 1 out]
        n308 = Index Array(array=w1451, index=1 ("Index")) -> (element=w1447:dbl)
        n309 = Index Array(array=w1451, index=0 ("Index")) -> (element=w1448:dbl)
        n310 = call "4155C Config I Stress.vi"("VISA session"=w1482, "IDG"=w1448, "VDG compliance"=w1447, "error in (no error)"=w1481, "Display on/off"=TRUE) -> ("dup VISA resource name"=w1484:refnum<visa-resource-name>, "error out"=w1483:errorcluster)
        n311 = Index Array(array=w1451, index=2 ("Index")) -> (element=w1449:dbl)
        n312 = String To Path(string=w1477) -> (path=w1467:path)
        n313 = call "4155C Apply Stress.vi"("error in (no error)"=w1483, "Duration"=w1449, "Emergency Stop"=w1462, "VISA resource name in"=w1484) -> ("error out"=w1460:errorcluster, "VISA Resource Name out"=w1458:refnum<visa-resource-name>)
        n314 = VISA Write(VISA resource name=w1458, write buffer=":DISP ON" ("write buffer (\"\")"), error in (no error)=w1460) -> (VISA resource name out=w1457:refnum<visa-resource-name>, error out=w1459:errorcluster)  [unwired: 1 out]
        n315 = call <vilib>:"compatOverwrite.vi"("overwrite (F)"=TRUE) -> ("overwrite?"=w1446:T7)
        n316 = Open/Create/Replace File(file path (use dialog)=w1467, error in=w1459, operation (0:open)=w1446) -> (refnum out=w1470:refnum<file>, error out=w1469:errorcluster)  [unwired: 3 in, 1 out]
        n317 = call "4155C Write array to file.vi"("Byte Stream File Refnum"=w1470, "Header"=string[] ["I stress completed successfully", ""], "error in (no error)"=w1469) -> ("dup refnum"=w1472:refnum<file>, "error out"=w1471:errorcluster)  [unwired: 2 in]
        n318 = Close File(refnum=w1472, error in=w1471) -> (error out=w1465:errorcluster)  [unwired: 1 out]
      }
      frame "vsu2pulse" {
        n319 = Number To Decimal String(number=w1504) -> (decimal integer string=w1539:string)  [unwired: 1 in]
        n320 = Concatenate Strings(w1524, "-vsu2-" ("Substring"), w1539, w1503, ".txt" ("Substring")) -> (w1537:string)
        n321 = Fract/Exp String To Number(string=w1536) -> (number=w1512:dbl[])  [unwired: 3 in, 1 out]
        n322 = String To Path(string=w1537) -> (path=w1528:path)
        n323 = Index Array(array=w1512, index=1 ("Index")) -> (element=w1511:dbl)
        n324 = Index Array(array=w1512, index=0 ("Index")) -> (element=w1509:dbl)
        n325 = call "4155C Config VSU2 Stress.vi"("error in (no error)"=w1541, "VSU2"=w1509, "Display on/off"=TRUE, "VISA session"=w1542) -> ("error out"=w1543:errorcluster, "dup VISA resource name"=w1544:refnum<visa-resource-name>)
        n326 = call "4155C Apply Stress.vi"("error in (no error)"=w1543, "Duration"=w1511, "Emergency Stop"=w1523, "VISA resource name in"=w1544) -> ("error out"=w1521:errorcluster, "VISA Resource Name out"=w1519:refnum<visa-resource-name>)
        n327 = VISA Write(VISA resource name=w1519, write buffer=":DISP ON" ("write buffer (\"\")"), error in (no error)=w1521) -> (VISA resource name out=w1518:refnum<visa-resource-name>, error out=w1520:errorcluster)  [unwired: 1 out]
        n328 = call <vilib>:"compatOverwrite.vi"("overwrite (F)"=TRUE) -> ("overwrite?"=w1508:T7)
        n329 = Open/Create/Replace File(file path (use dialog)=w1528, error in=w1520, operation (0:open)=w1508) -> (refnum out=w1531:refnum<file>, error out=w1530:errorcluster)  [unwired: 3 in, 1 out]
        n330 = call "4155C Write array to file.vi"("Byte Stream File Refnum"=w1531, "Header"=string[] ["VSU2 pulse completed successfully", ""], "error in (no error)"=w1530) -> ("dup refnum"=w1533:refnum<file>, "error out"=w1532:errorcluster)  [unwired: 2 in]
        n331 = Close File(refnum=w1533, error in=w1532) -> (error out=w1526:errorcluster)  [unwired: 1 out]
      }
      frame "sample-fpp" {
        w1575 = string[] ["Time /s", "Id VgVd /A", "Ig VgVd /A", "Vp1 VgVd /V", "Vp2 VgVd /V"] ("Header")
        w1579 = "%d" ("format string")
        n332 = Number To Decimal String(number=w1564) -> (decimal integer string=w1627:string)  [unwired: 1 in]
        n333 = Fract/Exp String To Number(string=w1624) -> (number=w1612:dbl[])  [unwired: 3 in, 1 out]
        n334 = Concatenate Strings(w1618, "-samplefpp-" ("Substring"), w1627, w1563, ".txt" ("Substring")) -> (w1625:string)
        n335 = String To Path(string=w1625) -> (path=w1587:path)
        n336 = Index Array(array=w1612, index=0 ("Index")) -> (element=w1573:dbl)
        n337 = Index Array(array=w1612, index=1 ("Index")) -> (element=w1572:dbl)
        n338 = Index Array(array=w1612, index=2 ("Index")) -> (element=w1620:dbl)
        n339 = Index Array(array=w1612, index=3 ("Index")) -> (element=w1610:dbl)
        n340 = call "4155C Config Sampling Measurements FPP.vi"("VISA session"=w1630, "Num Points"=w1620, "Vg"=w1573, "Display on/off"=TRUE, "Gate Compliance"=w1619, "Drain Compliance"=w1628, "Standby"="Standby", "error in (no error)"=w1629, "Timings"=w1617, "Vd"=w1572, "Sample time"=w1610) -> ("dup VISA resource name"=w1589:refnum<visa-resource-name>, "error out"=w1588:errorcluster)  [unwired: 3 in]
        n341 = Number To Decimal String(number=w1573) -> (decimal integer string=w1599:string)  [unwired: 1 in]
        n342 = call "4155C Take Sample FPP.vi"("VISA resource name in"=w1589, "error in (no error)"=w1588, "Emergency Stop"=w1590) -> ("Time"=w1594:dbl[], "Vp1"=w1604:dbl[], "VISA Resource Name out"=w1570:refnum<visa-resource-name>, "Ig"=w1592:dbl[], "Id"=w1593:dbl[], "Vp2"=w1602:dbl[], "error out"=w1591:errorcluster)  [unwired: 10 in]
        n343 = Insert Into Array(array=dbl[][] [] ("Input Array"), new element=w1594) -> (w1608:dbl[][])  [unwired: 2 in]
        n344 = Number To Decimal String(number=w1572) -> (decimal integer string=w1597:string)  [unwired: 1 in]
        n345 = Insert Into Array(array=w1608, new element=w1593) -> (w1607:dbl[][])  [unwired: 2 in]
        n346 = Concatenate Strings("(Vg = " ("Substring"), w1599, "V, Vd = " ("Substring"), w1597, "V)" ("Substring")) -> (w1595:string)
        n347 = Insert Into Array(array=w1607, new element=w1592) -> (w1606:dbl[][])  [unwired: 2 in]
        n348 = Insert Into Array(array=w1606, new element=w1604) -> (w1603:dbl[][])  [unwired: 2 in]
        n349 = Insert Into Array(array=w1603, new element=w1602) -> (w1571:dbl[][])  [unwired: 2 in]
        n350 = Transpose 2D Array(2D array=w1571) -> (transposed array=w1601:dbl[][])
        n351 = call <vilib>:"compatOverwrite.vi"("overwrite (F)"=TRUE) -> ("overwrite?"=w1568:T7)
        n352 = Open/Create/Replace File(file path (use dialog)=w1587, error in=w1591, operation (0:open)=w1568) -> (refnum out=w1584:refnum<file>, error out=w1585:errorcluster)  [unwired: 3 in, 1 out]
        n353 = Array To Spreadsheet String(array=w1575, 3:w1579) -> (spreadsheet string=w1581:string)  [unwired: 1 in]
        n354 = Search and Replace String(replace all?=TRUE ("replace all? (F)"), input string=w1581, search string="VgVd", replace string=w1595) -> (result string=w1577:string)  [unwired: 4 in, 3 out]
        n355 = Spreadsheet String To Array(format string=w1579, spreadsheet string=w1577, array type (2D Dbl)=w1575) -> (array=w1576:string[])  [unwired: 1 in]
        n356 = call "4155C Write array to file.vi"("Byte Stream File Refnum"=w1584, "Header"=w1576, "Data Array"=w1601, "error in (no error)"=w1585) -> ("dup refnum"=w1582:refnum<file>, "error out"=w1583:errorcluster)  [unwired: 1 in]
        n357 = Close File(refnum=w1582, error in=w1583) -> (error out=w1569:errorcluster)  [unwired: 1 out]
      }
      frame "resample-fpp" {
        w1663 = string[] ["Time /s", "Id VgVd /A", "Ig VgVd /A", "Vp1 VgVd /V", "Vp2 VgVd /V"] ("Header")
        w1667 = "%d" ("format string")
        n358 = Number To Decimal String(number=w1649) -> (decimal integer string=w1707:string)  [unwired: 1 in]
        n359 = Fract/Exp String To Number(string=w1704) -> (number=w1656:dbl[])  [unwired: 3 in, 1 out]
        n360 = Concatenate Strings(w1700, "-resamplefpp-" ("Substring"), w1707, w1650, ".txt" ("Substring")) -> (w1705:string)
        n361 = String To Path(string=w1705) -> (path=w1675:path)
        n362 = Index Array(array=w1656, index=0 ("Index")) -> (element=w1662:dbl)
        n363 = Index Array(array=w1656, index=1 ("Index")) -> (element=w1661:dbl)
        n364 = Number To Decimal String(number=w1662) -> (decimal integer string=w1685:string)  [unwired: 1 in]
        n365 = call "4155C Take Sample FPP.vi"("VISA resource name in"=w1658, "error in (no error)"=w1657, "Emergency Stop"=w1676) -> ("Time"=w1680:dbl[], "Vp1"=w1690:dbl[], "VISA Resource Name out"=w1660:refnum<visa-resource-name>, "Ig"=w1678:dbl[], "Id"=w1679:dbl[], "Vp2"=w1688:dbl[], "error out"=w1677:errorcluster)  [unwired: 10 in]
        n366 = Insert Into Array(array=dbl[][] [] ("Input Array"), new element=w1680) -> (w1694:dbl[][])  [unwired: 2 in]
        n367 = Number To Decimal String(number=w1661) -> (decimal integer string=w1683:string)  [unwired: 1 in]
        n368 = Insert Into Array(array=w1694, new element=w1679) -> (w1693:dbl[][])  [unwired: 2 in]
        n369 = Concatenate Strings("(Vg = " ("Substring"), w1685, "V, Vd = " ("Substring"), w1683, "V)" ("Substring")) -> (w1681:string)
        n370 = Insert Into Array(array=w1693, new element=w1678) -> (w1692:dbl[][])  [unwired: 2 in]
        n371 = Insert Into Array(array=w1692, new element=w1690) -> (w1689:dbl[][])  [unwired: 2 in]
        n372 = Insert Into Array(array=w1689, new element=w1688) -> (w1655:dbl[][])  [unwired: 2 in]
        n373 = call <vilib>:"compatOverwrite.vi"("overwrite (F)"=TRUE) -> ("overwrite?"=w1654:T7)
        n374 = Open/Create/Replace File(file path (use dialog)=w1675, error in=w1677, operation (0:open)=w1654) -> (refnum out=w1672:refnum<file>, error out=w1673:errorcluster)  [unwired: 3 in, 1 out]
        n375 = Array To Spreadsheet String(array=w1663, 3:w1667) -> (spreadsheet string=w1669:string)  [unwired: 1 in]
        n376 = Transpose 2D Array(2D array=w1655) -> (transposed array=w1687:dbl[][])
        n377 = Search and Replace String(replace all?=TRUE ("replace all? (F)"), input string=w1669, search string="VgVd", replace string=w1681) -> (result string=w1665:string)  [unwired: 4 in, 3 out]
        n378 = Spreadsheet String To Array(format string=w1667, spreadsheet string=w1665, array type (2D Dbl)=w1663) -> (array=w1664:string[])  [unwired: 1 in]
        n379 = call "4155C Write array to file.vi"("Byte Stream File Refnum"=w1672, "Header"=w1664, "Data Array"=w1687, "error in (no error)"=w1673) -> ("dup refnum"=w1670:refnum<file>, "error out"=w1671:errorcluster)  [unwired: 1 in]
        n380 = Close File(refnum=w1670, error in=w1671) -> (error out=w1659:errorcluster)  [unwired: 1 out]
      }
      frame "serial" {
        n381 = local read "Termination char\n(0xA = '\\n' = LF)\n(0xD = '\\r' = CR)"() -> (w1734:u8)
        n382 = local read "Enable Termination\nChar (T)"() -> (w1735:bool)
        n383 = Index Array(array=w1742, index=0 ("Index")) -> (element=w1741:string)
        n384 = local read "parity"() -> (w1725:u16)
        n385 = local read "Delay before read (ms)"() -> (w1736:u32)
        n386 = local read "byte count"() -> (w1733:u32)
        n387 = local read "Timeout (ms)"() -> (w1732:u32)
        n388 = local read "VISA resource name"() -> (w1729:refnum<visa-resource-name>)
        n389 = local read "baud rate"() -> (w1728:u32)
        n390 = local read "Serial End Mode for Reads"() -> (w1727:u16)
        n391 = local read "data bits"() -> (w1726:u16)
        n392 = local read "stop bits"() -> (w1731:u16)
        n393 = local read "flow control"() -> (w1730:u16)
        n394 = call "Serial write and read v0.5.vi"("Delay before read (ms)"=w1736, "Termination char\n(0xA = '\\n' = LF)\n(0xD = '\\r' = CR)"=w1734, "Enable Termination\nChar (T)"=w1735, "parity"=w1725, "stop bits"=w1731, "string to write"=w1741, "flow control"=w1730, "byte count"=w1733, "Serial Settings:Serial End Mode for Reads"=w1727, "Timeout (ms)"=w1732, "error in (no error)"=w1747, "VISA resource name"=w1729, "baud rate"=w1728, "data bits"=w1726) -> ("Serial port output"=w1737:string, "error out"=w1746:errorcluster)
        n395 = Build Array (concatenate)(w1737, w1738) -> (w1739:string[])
      }
      frame "pump" {
        # "Time array for valve position"
        # "Time array for absolute plunger position"
        # "Valve position"
        # "Absolute plunger position"
        # "Remove \"_\""
        # "Check if hard stop is pressed."
        # "Check if halt is pressed."
        # "Check if pump is idle. Else halt."
        n396 = Index Array(array=w1811, index=0 ("Index")) -> (element=w1788:string)
        n397 = case shown="\"No error\", Default" w1786 {
          tunnel: w1788 -> [w1847 _ w1849 w1850 w1851 w1852 _ _ w1855 w1856 _]
          tunnel: [w1847 "/1H" w1849 w1850 w1851 w1852 "/1H" "/1H" w1855 w1856 "/1H"] -> w1787
          frame "No error", Default {
          }
          frame "Initialization" {
          }
          frame "Invalid command" {
          }
          frame "Invalid operand" {
          }
          frame "Device not initialized" {
          }
          frame "Internal failure" {
          }
          frame "Plunger overload" {
          }
          frame "Valve overload" {
          }
          frame "Plunger move not allowed" {
          }
          frame "A/D converter failure" {
          }
          frame "Command overflow" {
          }
        }
        n398 = local read "Hard stop pump"() -> (w1790:bool)
        n399 = local read "Halt pump"() -> (w1793:bool)
        n400 = local read "Serial End Mode for Reads"() -> (w1799:u16)
        n401 = local read "flow control"() -> (w1802:u16)
        n402 = local read "stop bits"() -> (w1803:u16)
        n403 = local read "parity"() -> (w1797:u16)
        n404 = local read "Delay before read (ms)"() -> (w1808:u32)
        n405 = local read "byte count"() -> (w1805:u32)
        n406 = local read "Timeout (ms)"() -> (w1804:u32)
        n407 = local read "VISA resource name"() -> (w1801:refnum<visa-resource-name>)
        n408 = local read "baud rate"() -> (w1800:u32)
        n409 = local read "Enable Termination\nChar (T)"() -> (w1807:bool)
        n410 = local read "Termination char\n(0xA = '\\n' = LF)\n(0xD = '\\r' = CR)"() -> (w1806:u8)
        n411 = case shown="True" w1793 {
          tunnel: [w1861 "/1H"] -> w1792
          tunnel: w1787 -> [w1861 _]
          frame False {
          }
          frame True {
            n412 = local write "Halt pump"(FALSE) -> ()
          }
        }
        n413 = case shown="True" w1790 {
          tunnel: [w1858 "/1T"] -> w1791
          tunnel: w1792 -> [w1858 _]
          frame False {
          }
          frame True {
            n414 = local write "Hard stop pump"(FALSE) -> ()
          }
        }
        n415 = local read "data bits"() -> (w1798:u16)
        n416 = String Subset(string=w1782, offset (0)=1) -> (substring=w1780:string)  [unwired: 1 in]
        n417 = call "SPM Pump v0.6.vi"("Termination char\n(0xA = '\\n' = LF)\n(0xD = '\\r' = CR)"=w1806, "Enable Termination\nChar (T)"=w1807, "Timeout (ms)"=w1804, "Serial Settings:Serial End Mode for Reads"=w1799, "byte count"=w1805, "Delay before read (ms)"=w1808, "Time <input>"=w1785, "error in (no error)"=w1816, "Serial port input"=w1791, "VISA resource name"=w1801, "parity"=w1797, "baud rate"=w1800, "stop bits"=w1803, "data bits"=w1798, "flow control"=w1802, "Time units <input>"=w1780) -> ("Input command"=w1779:string, "Serial port data"=w1769:string[], "Pump status"=w1775:string, "Valve position"=w1777:i32, "Absolute plunger position"=w1789:i32, "Serial port"=w1784:string, "error out"=w1815:errorcluster)  [unwired: 1 in, 4 out]
        n418 = case shown="\"?6\"" w1779 {
          tunnel: [w1828 w1836 w1842] -> w1796
          tunnel: w1795 -> [w1828 w1835 w1842]
          tunnel: w1789 -> [_ w1834 _]
          tunnel: w1776 -> [w1827 w1833 w1843]
          tunnel: [w1827 w1833 w1845] -> w1778
          tunnel: w1777 -> [_ _ w1844]
          tunnel: w1774 -> [_ w1832 w1840]
          tunnel: w1773 -> [w1826 w1831 w1841]
          tunnel: [w1826 w1830 w1841] -> w1772
          tunnel: [w1825 w1829 w1839] -> w1771
          tunnel: w1770 -> [w1825 w1829 w1838]
          frame "Q", Default {
          }
          frame "?" {
            n419 = Build Array (concatenate)(w1835, w1834) -> (w1836:i32[])
            n420 = Build Array (concatenate)(w1831, w1832) -> (w1830:i32[])
            n421 = call "4155C Split array.vi"("X data in"=w1830, "Y1 data in"=w1836) -> ("Array of clusters"=w1837:cluster{"Y data in":dbl[], "X data in":dbl[]}[])  [unwired: 5 in, 1 out]
            n422 = local write "Absolute plunger position vs time"(w1837) -> ()
          }
          frame "?6" {
            n423 = Build Array (concatenate)(w1843, w1844) -> (w1845:i32[])
            n424 = Build Array (concatenate)(w1838, w1840) -> (w1839:i32[])
            n425 = call "4155C Split array.vi"("X data in"=w1839, "Y1 data in"=w1845) -> ("Array of clusters"=w1846:cluster{"Y data in":dbl[], "X data in":dbl[]}[])  [unwired: 5 in, 1 out]
            n426 = local write "Valve position vs time"(w1846) -> ()
          }
        }
        n427 = Build Array (concatenate)(w1767, w1769) -> (w1768:string[][])
        n428 = Build Array (concatenate)(w1783, w1784) -> (w1809:string[])
      }
    }
    n429 = Build Array(w124, w51, w61, w60, w59, w58, w57, w56, w55, w54, w53, w52, w50) -> (w167:dbl[][])
    n430 = Transpose 2D Array(2D array=w167) -> (transposed array=w166:dbl[][])
    n431 = Concatenate Strings(w102, "Prefix (Imax,Imin,Ion,Ioff)", "Suffix (Idmax-Idmin)") -> (w179:string)
    n432 = Build Array(w83, "Is max /A" ("VAR2 Name"), "Is min /A" ("VAR2 Name"), "Id max /A" ("VAR2 Name"), "Id min /A" ("VAR2 Name"), "Ig max /A" ("VAR2 Name"), "Ig min /A" ("VAR2 Name"), "Is on /A" ("VAR2 Name"), "Is off /A" ("VAR2 Name"), "Id on /A" ("VAR2 Name"), "Id off /A" ("VAR2 Name"), "Ig on /A" ("VAR2 Name"), "Ig off /A" ("VAR2 Name")) -> (w172:string[])
    n433 = Array To Spreadsheet String(array=w166, 3:"%e" ("format string")) -> (spreadsheet string=w170:string)  [unwired: 1 in]
    n434 = Array To Spreadsheet String(array=w172, 3:"" ("format string")) -> (spreadsheet string=w171:string)  [unwired: 1 in]
    n435 = String To Path(string=w179) -> (path=w178:path)
    n436 = Build Array(w171, w170) -> (w169:string[])
    n437 = Write to Text File(file (use dialog)=w178, text=w169, error in=w120) -> (refnum out=w180:refnum<file>, error out=w168:errorcluster)  [unwired: 1 in, 1 out]
    n438 = Close File(refnum=w180, error in=w168) -> (error out=w101:errorcluster)  [unwired: 1 out]
    n439 = Build Array(w97, w125) -> (w132:i32[][])
    n440 = Build Array(w83, "Absolute plunger position" ("VAR2 Name")) -> (w135:string[])
    n441 = Transpose 2D Array(2D array=w132) -> (transposed array=w123:i32[][])
    n442 = Array To Spreadsheet String(array=w135, 3:"" ("format string")) -> (spreadsheet string=w134:string)  [unwired: 1 in]
    n443 = Array To Spreadsheet String(array=w123, 3:"%e" ("format string")) -> (spreadsheet string=w131:string)  [unwired: 1 in]
    n444 = Build Array(w134, w131) -> (w137:string[])
    n445 = Concatenate Strings(w102, "Prefix (plunger)", "Suffix (plunger)") -> (w129:string)
    n446 = String To Path(string=w129) -> (path=w126:path)
    n447 = Write to Text File(file (use dialog)=w126, text=w137, error in=w101) -> (refnum out=w130:refnum<file>, error out=w139:errorcluster)  [unwired: 1 in, 1 out]
    n448 = Close File(refnum=w130, error in=w139) -> (error out=w100:errorcluster)  [unwired: 1 out]
    n449 = Concatenate Strings(w102, "Prefix (serial port log)", ".txt" ("Suffix")) -> (w147:string)
    n450 = String To Path(string=w147) -> (path=w144:path)
    n451 = Build Array(w83, "Serial port input" ("VAR2 Name"), "Pump status" ("VAR2 Name"), "Serial port output: ") -> (w87:string[])
    n452 = Array To Spreadsheet String(array=w93, 3:"" ("format string")) -> (spreadsheet string=w84:string)  [unwired: 1 in]
    n453 = Array To Spreadsheet String(array=w87, 3:"" ("format string")) -> (spreadsheet string=w85:string)  [unwired: 1 in]
    n454 = Build Array(w85, w84) -> (w86:string[])
    n455 = Array To Spreadsheet String(array=w92, 3:"" ("format string")) -> (spreadsheet string=w152:string)  [unwired: 1 in]
    n456 = Write to Text File(file (use dialog)=w144, text=w86, error in=w100) -> (refnum out=w148:refnum<file>, error out=w149:errorcluster)  [unwired: 1 in, 1 out]
    n457 = Close File(refnum=w148, error in=w149) -> (error out=w99:errorcluster)  [unwired: 1 out]
    n458 = local write "Serial port data"(w152) -> ()
    n459 = Build Array(w96, w104) -> (w112:i32[][])
    n460 = Build Array(w83, "Valve position" ("VAR2 Name")) -> (w115:string[])
    n461 = Transpose 2D Array(2D array=w112) -> (transposed array=w105:i32[][])
    n462 = Array To Spreadsheet String(array=w115, 3:"" ("format string")) -> (spreadsheet string=w114:string)  [unwired: 1 in]
    n463 = Array To Spreadsheet String(array=w105, 3:"%e" ("format string")) -> (spreadsheet string=w111:string)  [unwired: 1 in]
    n464 = Build Array(w114, w111) -> (w117:string[])
    n465 = Concatenate Strings(w102, "Prefix (valve)", "Suffix (valve)") -> (w109:string)
    n466 = String To Path(string=w109) -> (path=w106:path)
    n467 = Write to Text File(file (use dialog)=w106, text=w117, error in=w99) -> (refnum out=w110:refnum<file>, error out=w119:errorcluster)  [unwired: 1 in, 1 out]
    n468 = Close File(refnum=w110, error in=w119) -> (error out=w98:errorcluster)  [unwired: 1 out]
  }
  "error out" <- w9
